vi "AODScanner.vi"() -> ()   [LabVIEW 2014]
uses:
  AODAcq/AODAcq.lvclass
  <vilib>/DAQmx/write.llb/DAQmx Write (Analog DBL 1Chan 1Samp).vi
  <vilib>/DAQmx/read.llb/DAQmx Read (Analog Wfm 1Chan NSamp).vi
  <vilib>/DAQmx/miscellaneous.llb/DAQmx Fill In Error Info.vi
  Motion Stabilization/GlobalVars.vi
  <vilib>/Utility/error.llb/Error Cluster From Error Code.vi
  <vilib>/rvi/errors/niLvFpgaAdjustHostInterfaceError.vi
  <vilib>/rvi/interface/nirviMethod/nirviMethod.xnode
  FPGA_Control/AODRef.ctl
  FPGA Bitfiles/AodScanner_FPGATarget_AODControl(FPGA)_TyJc9yYmyGA.lvbitx
  <vilib>/rvi/interface/nirviReadWriteControl/nirviReadWriteControl.xnode
  <vilib>/FPGAPlugInAG/PXIe-7965R/niLvFpga_ReadFifo_PXIe-7965R.vi
  <vilib>/rvi/errors/niLvFpgaMergeErrorWithErrorCode.vi
  NiFpgaLv.dll
panel:
  in  "Add":bool=TRUE
  out "ZOut um":dbl
  out "YOut um":dbl
  out "XOut um":dbl
  in  "Reset AOD Cum Offsets":bool
  out "Cum AOD Offset Z":dbl
  out "Cum AOD Offset X":dbl
  out "Cum AOD Offset Y":dbl
  in  "Noise Frequency (Hz)":dbl=0.1
  in  "Noise Amplitude (um)":dbl=3.0
  in  "Simulate Scanning Noise":bool
  in  "Invert Intensity":bool
  in  "AOD Feedback":bool
  out "XOut":i32
  out "ZOut":i32
  out "YOut":i32
  in  "Invert Z":bool=TRUE
  in  "Invert X":bool
  in  "Invert Y":bool=TRUE
  in  "Scan Offset X":dbl format="%#_13g"
  in  "Scan Offset Y":dbl format="%#_13g"
  in  "Scan Offset Z":dbl format="%#_13g"
  in  "Set AOD Scan Offset":bool
  out "globals_semaphore":T1
  out "Scan Settings Saved":T2
  out "y_scale":dbl
  out "x_scale":dbl
  out "Motion Points (Ch1)":u32
  in  "Per Cell Motion Analysis":bool
  in  "Sampling Structure":u16(ring) items=["Cube Vertices"]
  out "EventDone":bool
  in  "ForcePointScan":bool
  out "Selection":u32
  in  "ForceVolumeScan":bool
  out "Scan Settings (um) Saved":T2={"XStart"=-100, "XEnd"=100, "XNum"=250, "YStart"=-100, "YEnd"=100, "YNum"=250, "ZStart"=-30, "ZEnd"=70, "ZNum"=60}
  out "Motion FIFO":refnum<queue>
  out "Points_um":dbl[][](array[numeric])
  out "Stopped":bool
  in  "Power":dbl(slide)=2.5 min=0.0 max=5.0 step=0.1 scale=0.0..2.5
  in  "Debug":bool
  out "Number of Motion Planes":i32
  out "Motion Plane Centers":i32[][](array[numeric])
  in  "GridPoints":u16=10
  out "X-Y Motion Points":i32[][](array[numeric])
  out "Y-Z Motion Points":i32[][](array[numeric])
  out "error out":errorcluster
  out "error out 2":errorcluster
  in  "External Magnification":dbl=1.3
  in  "Matlab Server IP Address":string="10.21.16.18"
  in  "Matlab Server Shared Folder":string="c:\\temp"
  out "Histogram":dynamicdata(graph)
  out "ROIs":T3(array[cluster])
  out "Motion ROIs":T3(array[cluster])
  out "Waveform Chart":waveform(dbl)(graph)
  out "Ephys":bool
  in  "Points":i32[][](array[numeric])
  in  "Abort":bool
  out "ScanProgress":dbl(slide) scale=0.0..1.0
  in  "Simulated Motion Signal":bool
  in  "TraceElements":u32=10000
  out "Out Points":i32[][](array[numeric])
  in  "Tab Control":enum32{"Setup", "Volume", "Traces", "Motion"}(tab)
  in  "AOD Correction Threshold":dbl=0.25
  in  "AOD Feedback Gain":dbl=0.5
  in  "Average Motion Channels":bool
  in  "LoadAODVolume":bool
  in  "AOD Correction Refractory Time":dbl=1.0
  in  "Motor Correction Threshold":dbl=2.0 format="%#_13g"
  in  "Motion Tracking":bool
  in  "Auto Recentering":bool
  in  "XNum":i32=100
  in  "YNum":i32=100
  in  "Onset (fraction)":dbl=0.99 format="%#_13g"
  in  "Offset (fraction)":dbl=0.01 format="%#_13g"
  in  "Post Recentering Wait (ms)":u32=1000
  in  "Store Raw":bool
  in  "Disp Volume":bool=TRUE
  in  "Save Volume":bool
  in  "Ephys Acq":bool
  in  "Motion rate (Hz)":dbl=10.0
  in  "Scan Settings (um)":T2={"XStart"=-100, "XEnd"=100, "XNum"=250, "YStart"=-100, "YEnd"=100, "YNum"=250, "ZStart"=-30, "ZEnd"=70, "ZNum"=60}
  in  "Objective":enum16{"20x Olympus"}(ring)
  in  "Scan Time (s)":dbl=3000.0
  in  "Volume Reps":i32=1 min=1 max=10000
  in  "Volume Scan":bool
  in  "Points Scan":bool
  in  "Motion Channel To Analyze":i32=1 min=1 max=2
  in  "Motion Analysis":bool
  in  "Auto Motion Plane Params":T4={"Z Offset Per Box (um)"=3, "Box Size (um)"=16.0}
  in  "Mirror Ch1 Display":bool
  in  "ClearMotionCenters":bool
  in  "Point Centering":bool=TRUE
  in  "Recenter":bool caption="OK Button"
  out "Cells Selected":u32
  in  "Contrast":dbl(slide)=99.63636363636364 scale=98.0..100.0
  out "ImCh2":T5(plugin-control)
  out "ImCh1":T5(plugin-control)
  in  "Section":dbl min=0.0 max=59.0 step=1.0
  in  "Segment":bool
  out "Motion Increment":u32
  in  "Offset":dbl(slide)=0.010101010101010102 scale=0.0..1.0
  in  "ClearPoints":bool
  out "Total Motion Points":i32
  out "Number of Motion Volumes":i32
  out "Motion Ch1":T5(plugin-control)
  out "Ephys Signals":waveform(dbl)[](graph)
  in  "Baseline Offset":dbl
  in  "Decimate":bool
  in  "Spacing":dbl=100.0
  out "Traces":waveform(dbl)[](graph)
  in  "Down Rate":i32=500
  out "Elements In Traces Queue":i32
  out "Progress":dbl(slide) scale=0.0..1.0
  out "Scan Settings":T2
  in  "VolumeElements":u32=10000
  out "Recording File":path
  out "Objective Position":cluster{"X":dbl, "Y":dbl, "Z":dbl}
  out "Lens Magnification":i32=20
  out "Finished":bool
  out "Image samples remaining":u32
  out "Motion samples remaining":u32
  out "Temporal samples remaining":u32
  out "Raw samples remaining":u32
  in  "stop":bool
  out "AODAcq out":refnum<class "AODAcq.lvclass">
  out "Volume":bool
  out "Scan":bool
  in  "SweepSettings":bool
  out "Numeric":i32=299
  # "On"
  # "Off"
  # "um"
  # "sec"
  # "um"
  # "Motor"
  # "AOD+Motor"
  # "Off"
  # "On"
  # "Volume Resolution (points)"
  # "Behavior Pause"
  # "Off"
  # "On"
  # "Off"
  # "On"
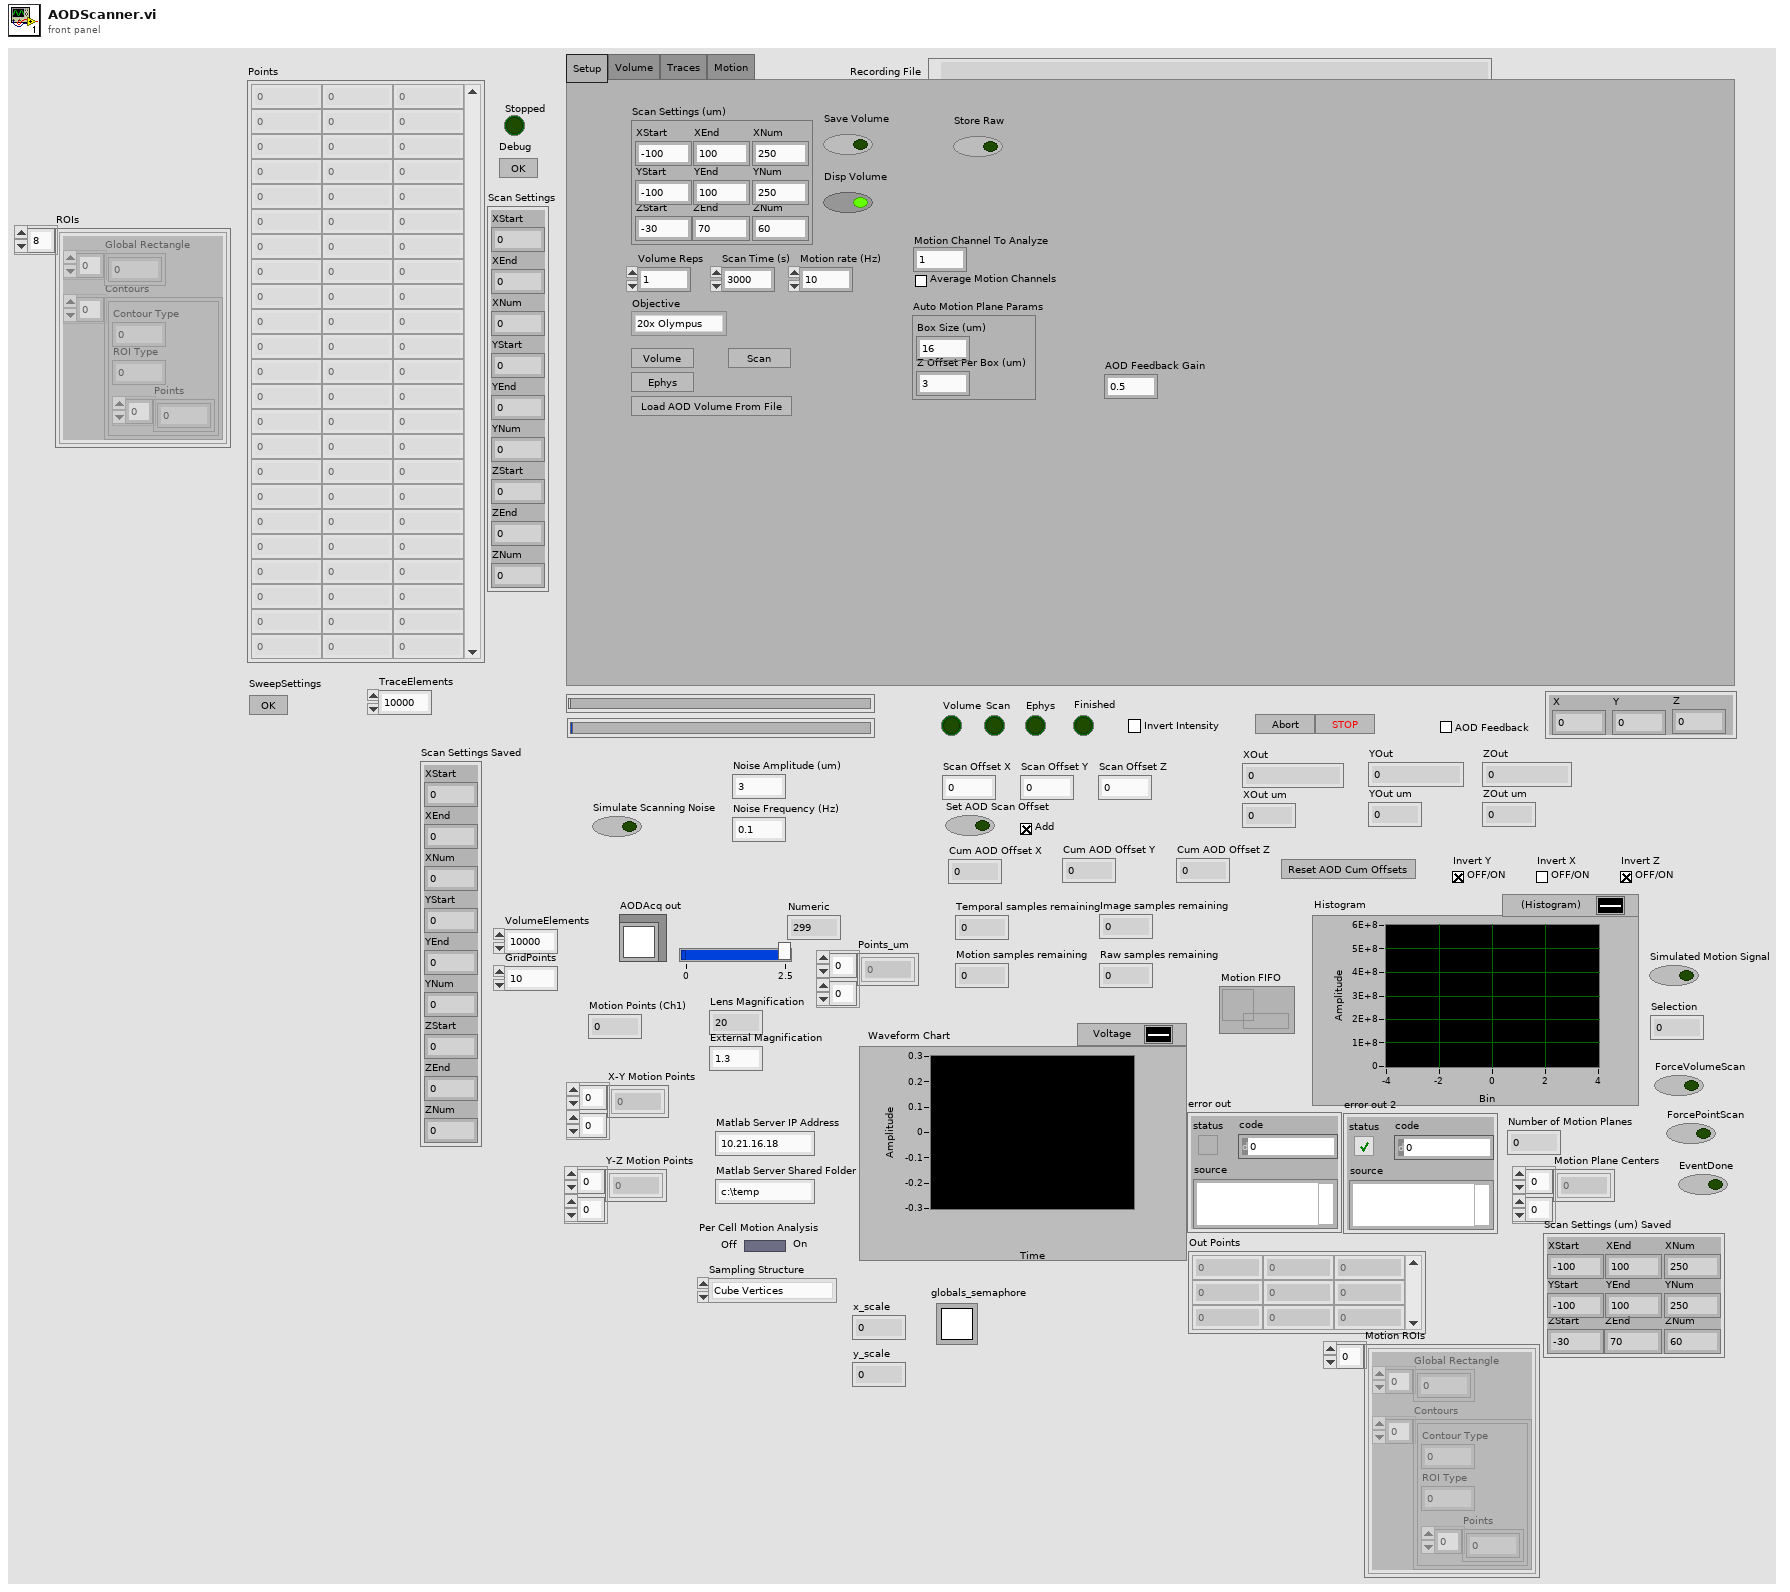
[diagram p1: front panel]
types:
  T1 = typedef "Semaphore RefNum" = refnum<k1>
  T2 = cluster{"XStart":i32, "XEnd":i32, "XNum":i32, "YStart":i32, "YEnd":i32, "YNum":i32, "ZStart":i32, "ZEnd":i32, "ZNum":i32}
  T3 = cluster{"Global Rectangle":i32[], "Contours":cluster{"Contour Type":u32, "ROI Type":u32, "Points":i32[]}[]}[]
  T4 = cluster{"Z Offset Per Box (um)":i32, "Box Size (um)":dbl}
  T5 = typedef "IMAQ Image.ctl" = refnum<image>
  T6 = cluster{"gridsize":u16, "data":i32[][], "coordinates":i32[][], "settings":i32[], "settings_um":i32[], "needsreference":bool}
  T7 = typedef "Image Type" = u32
  T8 = cluster{"Global Rectangle":i32[], "Contours":cluster{"Contour Type":u32, "ROI Type":u32, "Points":i32[]}[]}
  T9 = enum16{"big-endian, network order", "native, host order", "little-endian"}
  T10 = enum16{"open", "replace", "create", "open or create", "replace or create", "replace or create with confirmation"}
  T11 = cluster{"queue out":refnum<queue>, "queue out":refnum<queue>, "queue out":refnum<queue>, "queue out":refnum<queue>}
  T12 = typedef "AODRef.ctl" = refnum<k20>
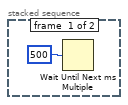
[diagram p2: hidden frame]
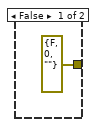
[diagram p4: hidden frame]
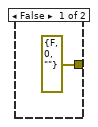
[diagram p5: hidden frame]
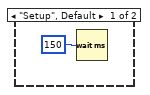
[diagram p6: hidden frame]
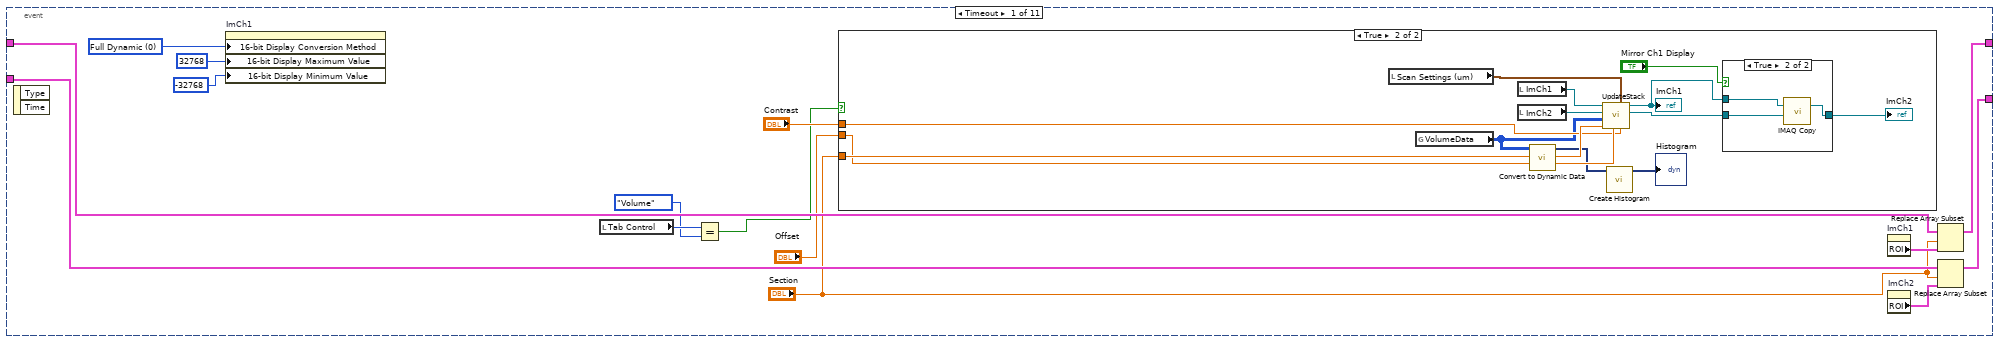
[diagram p8: hidden frame]
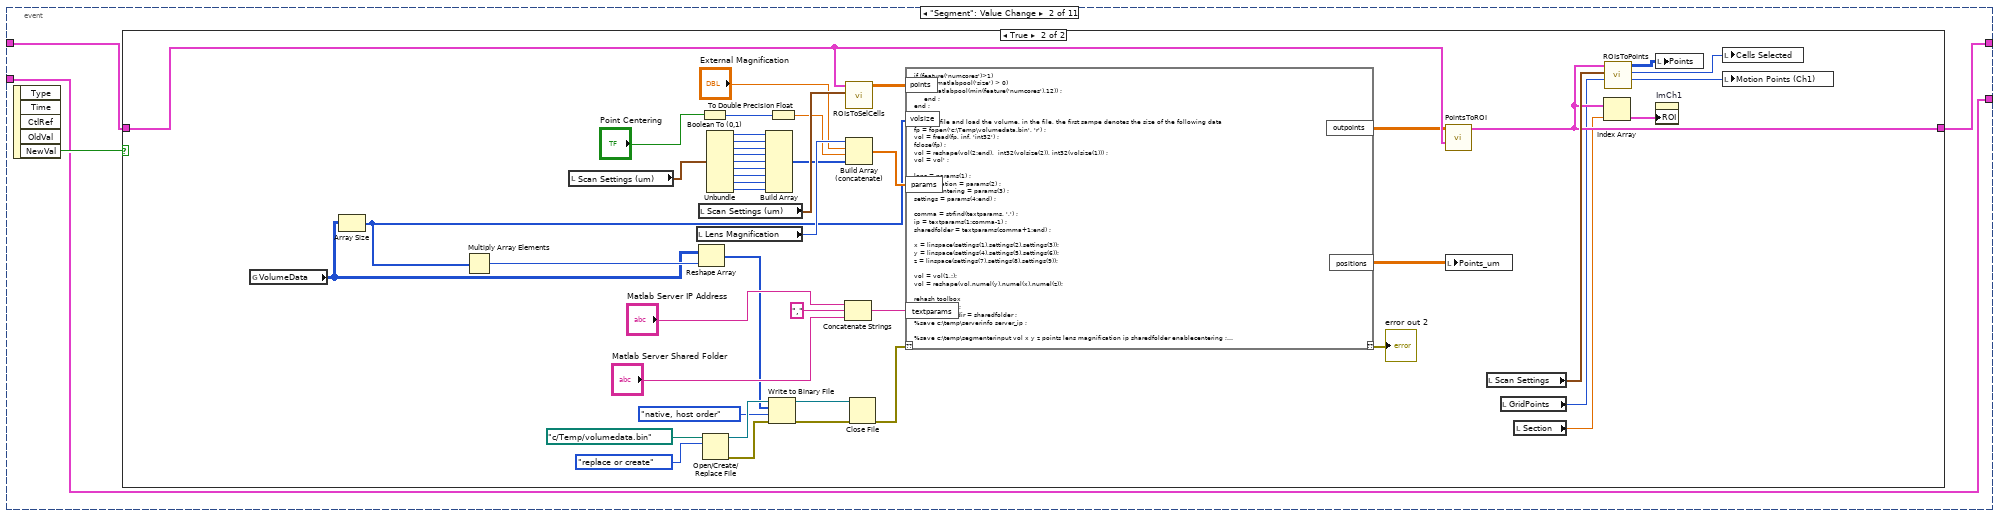
[diagram p11: hidden frame]
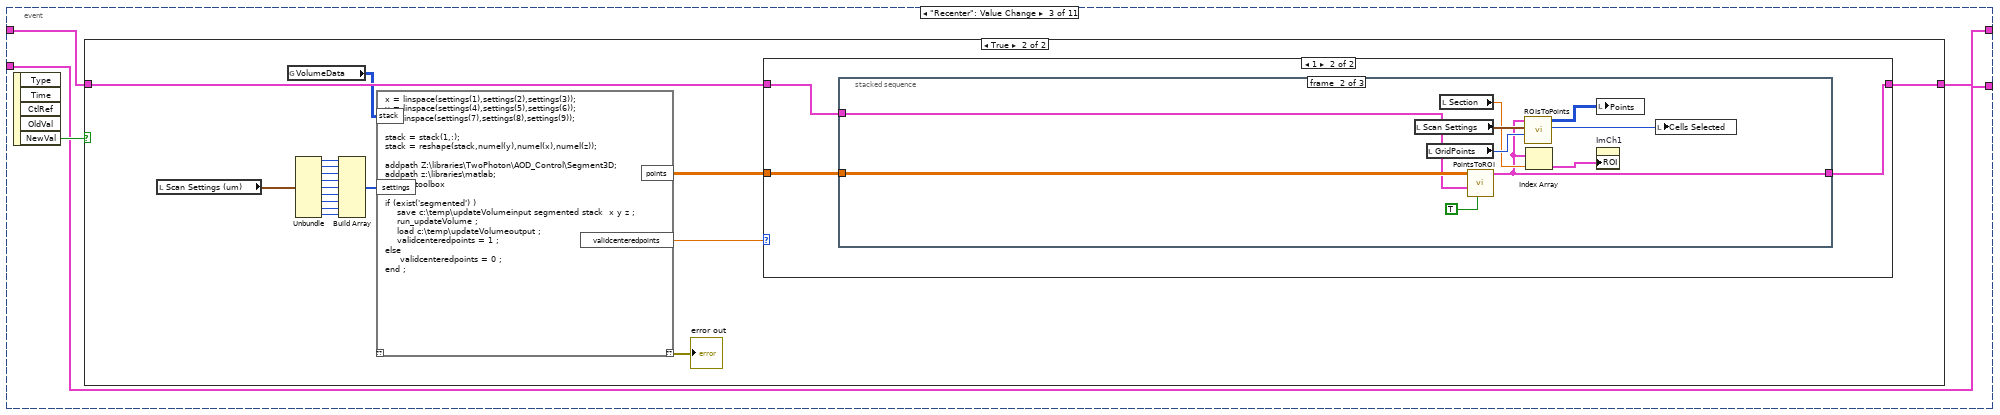
[diagram p13: hidden frame]
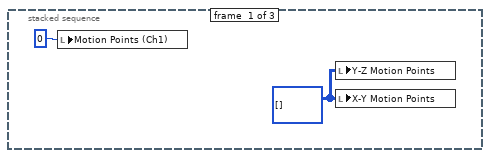
[diagram p16: hidden frame]
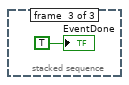
[diagram p17: hidden frame]
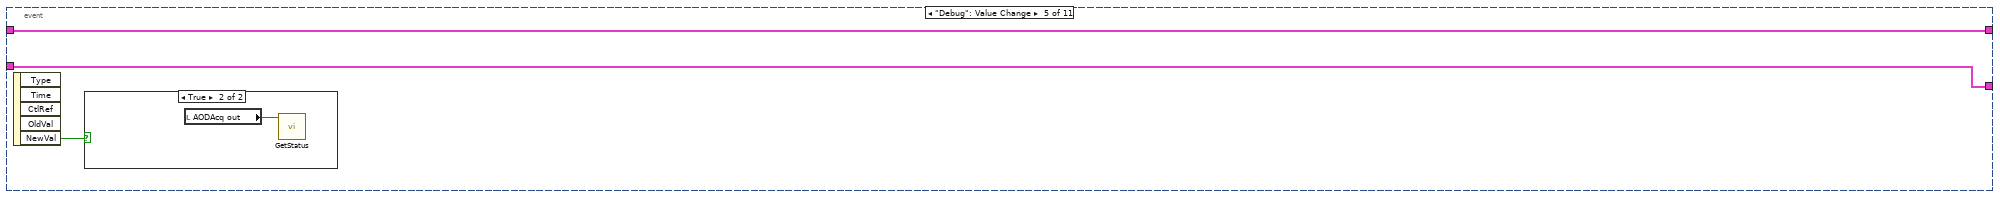
[diagram p19: hidden frame]
diagram:
  w11 = FALSE ("ForceVolumeScan")
  w27 = 100 ("max queue size (-1, unlimited)")
  w32 = T7 2 items=["Grayscale (U8)", "Grayscale (I16)", "Grayscale (SGL)", "Complex (CSG)", "RGB (U32)", "HSL (U32)", "RGB (U64)", "Grayscale (U16)"] ("Image Type")
  w9 = waveform(i32)[] []
  w42 = T7 0 items=["Grayscale (U8)", "Grayscale (I16)", "Grayscale (SGL)", "Complex (CSG)", "RGB (U32)", "HSL (U32)", "RGB (U64)", "Grayscale (U16)"] ("Image Type")
  w18 = T8 {"Global Rectangle"=[], "Contours"=[]} ("ROI")
  w52 = refnum<k21> "AOD Gain"  # DAQmx Global Channel
  n1 = local read "Scan Settings (um)"() -> (w46:T2)
  n2 = local write "ForceVolumeScan"(w11) -> ()
  n3 = local write "ForcePointScan"(w11) -> ()
  n4 = local write "Stopped"(FALSE ("Stopped")) -> ()
  n5 = local write "Stopped"(FALSE ("Stopped")) -> ()
  n6 = global write "GlobalVars.vi" "VI Open"(FALSE ("VI Open")) -> ()
  n7 = local write "Tab Control"(enum32{"Setup", "Volume", "Traces", "Motion"}."Setup" ("Tab Control")) -> ()
  n8 = Obtain Notifier(name (unnamed)="GoMove", notification data type="") -> (notifier out=w2:refnum<notifier>)  [unwired: 2 in, 2 out]
  n9 = Reciprocal(x="Motion rate (Hz)") -> (1/x=w20:dbl)
  n10 = global write "GlobalVars.vi" "Sampling Interval (sec)"(w20) -> ()
  n11 = global write "GlobalVars.vi" "GoMove Notifier"(w2) -> ()
  n12 = call <vilib>:"DAQmx Create Task.vi"("global virtual channels"=w52) -> ("task out"=w51:refnum<k21>, "error out"=w50:errorcluster)  [unwired: 4 in, 9 out]
  n13 = call "IMAQ Create"("Image Name"="Im1", "Image Type"=w42) -> ("New Image"=w54:T5)  [unwired: 3 in, 1 out]
  n14 = call "IMAQ Create"("Image Name"="Im2", "Image Type"=w42) -> ("New Image"=w53:T5)  [unwired: 3 in, 1 out]
  n15 = Unbundle By Name(w46) -> ("ZNum"=w17:i32)
  n16 = call "IMAQ Create"("Image Name"="Mot1", "Image Type"=w32) -> ("New Image"=→"Motion Ch1":T5)  [unwired: 3 in, 1 out]
  n17 = while {
    tunnel: w51 -> [w63]
    tunnel: w50 -> [w62]
    tunnel: [w61] -> w49
    tunnel: [w60] -> w48
    stop <- w59 stop-if-true
    n18 = Wait (ms)(milliseconds to wait=u32 1000) -> ()  [unwired: 1 out]
    n19 = local read "Stopped"() -> (w59:bool)
    n20 = call-poly <vilib>:"DAQmx Write.vi"("task/channels in"=w63, "data"="Power", "error in"=w62) -> ("task out"=w61:refnum<k21>, "error out"=w60:errorcluster)  [unwired: 10 in, 1 out]
  }
  n21 = local write "ImCh1"(w54) -> ()
  n22 = local write "ImCh2"(w53) -> ()
  n23 = Obtain Queue(max queue size (-1, unlimited)=w27, element data type=waveform(i32)[] []) -> (queue out=w38:refnum<queue>)  [unwired: 3 in, 2 out]
  n24 = Obtain Queue(max queue size (-1, unlimited)=w27, element data type=waveform(dbl)[] []) -> (queue out=w39:refnum<queue>)  [unwired: 3 in, 2 out]
  n25 = Obtain Queue(max queue size (-1, unlimited)=w27, element data type=w9) -> (queue out=w37:refnum<queue>)  [unwired: 3 in, 2 out]
  n26 = Obtain Queue(element data type=w9) -> (queue out=w8:refnum<queue>)  [unwired: 4 in, 2 out]
  n27 = call <vilib>:"Obtain Semaphore Reference.vi"("name (unnamed)"="globals") -> ("error out"=w5:errorcluster, "semaphore"=w6:T1)  [unwired: 4 in, 1 out]
  "globals_semaphore" <- w6
  n28 = Obtain Queue(name (unnamed)="Motion FIFO", element data type=0) -> (queue out=w13:refnum<queue>)  [unwired: 3 in, 2 out]
  "Motion FIFO" <- w13
  n29 = Obtain Queue(max queue size (-1, unlimited)=100, name (unnamed)="MotionAnalysis", element data type=T6 {"gridsize"=0, "data"=[], "coordinates"=[], "settings"=[], "settings_um"=[], "needsreference"=FALSE}) -> (queue out=w1:refnum<queue>)  [unwired: 2 in, 2 out]
  n30 = Decrement(x=w17) -> (x-1=w41:i32)
  n31 = Initialize Array(w18, w17) -> (w45:T3)
  n32 = Initialize Array(w18, w17) -> (w16:T3)
  n33 = while {
    shift-right: [w66] -> _
    shift-left: w45 -> [w70]
    shift-right: [w65] -> _
    shift-left: w16 -> [w67]
    stop <- w68 stop-if-true
    n34 = event shown="[3] \"Invert Intensity\": Value Change" {
      selector: _ -> [_ _ _ _ _ _ _ _ _ _ _]
      dyn-events: _ -> [_ _ _ _ _ _ _ _ _ _ _]
      timeout: 200 -> [_ _ _ _ _ _ _ _ _ _ _]
      tunnel: w70 -> [w84 w105 w156 w195 w202 w211 w239 w240 w253 w257 w269]
      tunnel: [w85 w104 w157 w195 w202 w211 w236 w240 w252 w258 w269] -> w66
      tunnel: [w72 w103 w155 w194 w201 w206 w228 w241 w249 w256 w270] -> w65
      tunnel: w67 -> [w75 w103 w155 w194 w201 w206 w228 w246 w251 w256 w268]
      event Timeout {
        w80 = u32 0 items=["Full Dynamic", "Downshift", "Given Range", "90% Dynamic", "Given Percent Range"] ("16-bit Display Mapping:Conversion Method")
        n35 = event-data() -> ()  [unwired: 1 in, 2 out]
        n36 = property on="ImCh1" class="ImageControl"("16-bit Display Conversion Method"=w80, "16-bit Display Maximum Value"=32768 ("16-bit Display Mapping:Maximum Value"), "16-bit Display Minimum Value"=-32768 ("16-bit Display Mapping:Maximum Value")) -> ()  [unwired: 2 in, 2 out]
        n37 = local read "Tab Control"() -> (w82:enum32{"Setup", "Volume", "Traces", "Motion"})
        n38 = Equal?(x=w82, y=enum32{"Setup", "Volume", "Traces"}."Volume") -> (x = y?=w71:bool)
        n39 = case shown="True" w71 {
          tunnel: "Section" -> [_ w95]
          tunnel: "Offset" -> [_ w94]
          tunnel: "Contrast" -> [_ w93]
          frame False {
          }
          frame True {
            n40 = local read "Scan Settings (um)"() -> (w96:T2)
            n41 = global read "GlobalVars.vi" "VolumeData"() -> (w86:i32[][])
            n42 = local read "ImCh1"() -> (w98:T5)
            n43 = local read "ImCh2"() -> (w97:T5)
            n44 = call "Convert to Dynamic Data"("2D Array"=w86) -> ("Dynamic Data Type"=w92:dynamicdata)  [unwired: 3 in]
            n45 = call "UpdateStack.vi"("Contrast"=w93, "Scan Settings"=w96, "Offset"=w94, "Section"=w95, "ImData"=w86, "Im2 2"=w97, "Im1 In"=w98) -> ("Im2 Out"=w87:T5, "Im1 Out"=w89:T5)  [unwired: 3 in]
            "ImCh1" <- w89
            n46 = call "Create Histogram"("Signal"=w92) -> ("Histogram"=→"Histogram":dynamicdata)  [unwired: 9 in, 1 out]
            n47 = case shown="True" "Mirror Ch1 Display" {
              tunnel: w89 -> [_ w101]
              tunnel: [w99 w100] -> w88
              tunnel: w87 -> [w99 w102]
              frame False {
              }
              frame True {
                n48 = call "IMAQ Copy"("Image Dst"=w102, "Image Src"=w101) -> ("Image Dst Out"=w100:T5)  [unwired: 4 in, 1 out]
              }
            }
            "ImCh2" <- w88
          }
        }
        n49 = property on="ImCh1" class="ImageControl"() -> ("ROI"=w83:T8)  [unwired: 2 in, 2 out]
        n50 = property on="ImCh2" class="ImageControl"() -> ("ROI"=w74:T8)  [unwired: 2 in, 2 out]
        n51 = Replace Array Subset(array=w84, new element=w83, index="Section") -> (w85:T3)
        n52 = Replace Array Subset(array=w75, new element=w74, index="Section") -> (w72:T3)
      }
      event "Segment": Value Change {
        n53 = event-data() -> ("NewVal"=w106:bool)  [unwired: 1 in, 4 out]
        n54 = case shown="True" w106 {
          tunnel: w105 -> [w107 w137]
          tunnel: [w107 w141] -> w104
          frame False {
          }
          frame True {
            n55 = global read "GlobalVars.vi" "VolumeData"() -> (w108:i32[][])
            n56 = Array Size(array=w108) -> (size(s)=w110:i32[])
            n57 = Multiply Array Elements(1:w110) -> (0:w117:i32)
            n58 = local read "Scan Settings (um)"() -> (w154:T2)
            n59 = local read "Lens Magnification"() -> (w133:i32)
            n60 = local read "Scan Settings (um)"() -> (w135:T2)
            n61 = Reshape Array(w108, w117) -> (w115:i32[])
            n62 = Boolean To (0,1)(Boolean="Point Centering") -> (0, 1=w138:i16)
            n63 = Open/Create/Replace File(file path (use dialog)=path "c:/Temp/volumedata.bin", operation (0:open)=T10."replace or create") -> (refnum out=w116:refnum<file>, error out=w114:errorcluster)  [unwired: 4 in, 1 out]
            n64 = Unbundle(w154) -> ("XStart"=w153:i32, "XEnd"=w152:i32, "XNum"=w151:i32, "YStart"=w150:i32, "YEnd"=w149:i32, "YNum"=w148:i32, "ZStart"=w147:i32, "ZEnd"=w146:i32, "ZNum"=w145:i32)
            n65 = Build Array(w153, w152, w151, w150, w149, w148, w147, w146, w145) -> (w127:i32[])
            n66 = Write to Binary File(file (use dialog)=w116, data=w115, error in=w114, 9:T9."native, host order" ("byte order (0:big-endian, network order)")) -> (refnum out=w112:refnum<file>, error out=w113:errorcluster)  [unwired: 2 in, 1 out]
            n67 = To Double Precision Float(number=w138) -> (double precision float=w131:dbl)
            n68 = Concatenate Strings("Matlab Server IP Address", "," ("string"), "Matlab Server Shared Folder") -> (w122:string)
            n69 = call "ROIsToSelCells.vi"("Scan Settings"=w135, "ROI"=w137) -> ("Points_um"=w134:dbl[][])  [unwired: 8 in, 1 out]
            n70 = Build Array (concatenate)(w133, "External Magnification", w131, w127) -> (w126:dbl[])
            n71 = Close File(refnum=w112, error in=w113) -> (error out=w111:errorcluster)  [unwired: 1 out]
            n72 = script code="if (feature('numcores')>1)\n     if (~matlabpool('size') > 0)\n         matlabpool(min(feature('numcores'),12)) ;\n     end ;\nend ;\n\n% open file and load the volume, in the file, the first sampe denotes the size of the following data\nfp = fopen('c:\\Temp\\volumedata.bin', 'r') ;\nvol = fread(fp, inf, 'int32') ;\nfclose(fp) ;\nvol = reshape(vol(2:end),  int32(volsize(2)), int32(volsize(1))) ;\nvol = vol' ;\n\nlens = params(1) ;\nmagnification = params(2) ;\nenablecentering = params(3) ;\nsettings = params(4:end) ;\n\ncomma = strfind(textparams, ',') ;\nip = textparams(1:comma-1) ;\nsharedfolder = textparams(comma+1:end) ;\n\nx = linspace(settings(1),settings(2),settings(3));\ny = linspace(settings(4),settings(5),settings(6));\nz = linspace(settings(7),settings(8),settings(9));\n\nvol = vol(1,:);\nvol = reshape(vol,numel(y),numel(x),numel(z));\n\nrehash toolbox\nserver_ip = ip ;\nserver_shareddir = sharedfolder ;\n%save c:\\temp\\serverinfo server_ip ;\n\n%save c:\\temp\\segmenterinput vol x y z points lens magnification ip sharedfolder enablecentering ;\n%remote_run_segmenter ;\nseg = aod.Segmenter(vol, x, y, z, points, lens, magnification, ip, sharedfolder, enablecentering ) ;\nsegmented = SegmenterDisplay(seg) ;\n\nfilename = sprintf('%s\\\\seg.mat', sharedfolder) ;\nload(filename) ;\npoints = centered_coordinates;\npositions = points; % in microns\n\n% Need to convert points into indicies into the array\nfor i = 1:size(points,1)\n   [~,idx] = min(abs(points(i,1)-x)); points(i,1) = idx;\n   [~,idx] = min(abs(points(i,2)-y)); points(i,2) = idx;\n   [~,idx] = min(abs(points(i,3)-z)); points(i,3) = idx;\nend\noutpoints = points ;"("??"=w111, "params"=w126, "textparams"=w122, "points"=w134, "volsize"=w110) -> ("??"=→"error out 2":errorcluster, "outpoints"=w121:dbl[][], "positions"=w120:dbl[][])
            n73 = call "PointsToROI.vi"("Old ROIs"=w137, "Points"=w121) -> ("ROIs"=w141:T3)  [unwired: 9 in]
            n74 = local write "Points_um"(w120) -> ()
            n75 = local read "Scan Settings"() -> (w143:T2)
            n76 = local read "GridPoints"() -> (w136:u16)
            n77 = local read "Section"() -> (w140:dbl)
            n78 = Index Array(array=w141, index=w140) -> (element=w142:T8)
            n79 = call "ROIsToPoints.vi"("GridPoints"=w136, "Scan Settings"=w143, "ROI"=w141) -> ("Number of motion points"=w124:i32, "Number of points"=w144:i32, "Points"=w123:i32[][])  [unwired: 4 in, 2 out]
            n80 = local write "Points"(w123) -> ()
            n81 = property on="ImCh1" class="ImageControl"("ROI"=w142) -> ()  [unwired: 2 in, 2 out]
            n82 = local write "Cells Selected"(w144) -> ()
            n83 = local write "Motion Points (Ch1)"(w124) -> ()
          }
        }
      }
      event "Recenter": Value Change {
        n84 = event-data() -> ("NewVal"=w158:bool)  [unwired: 1 in, 4 out]
        n85 = case shown="True" w158 {
          tunnel: [w159 w163] -> w157
          tunnel: w156 -> [w159 w164]
          frame False {
          }
          frame True {
            n86 = local read "Scan Settings (um)"() -> (w165:T2)
            n87 = global read "GlobalVars.vi" "VolumeData"() -> (w160:i32[][])
            n88 = Unbundle(w165) -> ("XStart"=w176:i32, "XEnd"=w175:i32, "XNum"=w174:i32, "YStart"=w173:i32, "YEnd"=w172:i32, "YNum"=w171:i32, "ZStart"=w170:i32, "ZEnd"=w169:i32, "ZNum"=w168:i32)
            n89 = Build Array(w176, w175, w174, w173, w172, w171, w170, w169, w168) -> (w167:i32[])
            n90 = script code="x = linspace(settings(1),settings(2),settings(3));\ny = linspace(settings(4),settings(5),settings(6));\nz = linspace(settings(7),settings(8),settings(9));\n\nstack = stack(1,:);\nstack = reshape(stack,numel(y),numel(x),numel(z));\n\naddpath Z:\\libraries\\TwoPhoton\\AOD_Control\\Segment3D;\naddpath z:\\libraries\\matlab;\nrehash toolbox\n\nif (exist('segmented') )\n    save c:\\temp\\updateVolumeinput segmented stack  x y z ;\n    run_updateVolume ;\n    load c:\\temp\\updateVolumeoutput ;\n    validcenteredpoints = 1 ;\nelse\n     validcenteredpoints = 0 ;\nend ;"("stack"=w160, "settings"=w167) -> ("??"=→"error out":errorcluster, "points"=w166:dbl[][], "validcenteredpoints"=w162:dbl)  [unwired: 1 in]
            n91 = case shown="1" w162 {
              tunnel: w166 -> [_ w180]
              tunnel: w164 -> [w177 w179]
              tunnel: [w177 w178] -> w163
              frame 0, Default {
              }
              frame 1 {
                n92 = stacked-sequence {
                  tunnel: w180 -> [_ w192 _]
                  tunnel: w179 -> [_ w188 _]
                  tunnel: [_ w185 _] -> w178
                  frame #0 {
                    w181 = i32[][] [] ("Points")
                    n93 = local write "Motion Points (Ch1)"(u32 0 ("Number of Motion Points")) -> ()
                    n94 = local write "Y-Z Motion Points"(w181) -> ()
                    n95 = local write "X-Y Motion Points"(w181) -> ()
                  }
                  frame #1 {
                    n96 = local read "Scan Settings"() -> (w189:T2)
                    n97 = local read "GridPoints"() -> (w190:u16)
                    n98 = local read "Section"() -> (w186:dbl)
                    n99 = call "PointsToROI.vi"("Clear Motion Planes"=TRUE, "Old ROIs"=w188, "Points"=w192) -> ("ROIs"=w185:T3)  [unwired: 8 in]
                    n100 = call "ROIsToPoints.vi"("GridPoints"=w190, "Scan Settings"=w189, "ROI"=w185) -> ("Number of points"=w191:i32, "Points"=w184:i32[][])  [unwired: 4 in, 3 out]
                    n101 = Index Array(array=w185, index=w186) -> (element=w187:T8)
                    n102 = local write "Points"(w184) -> ()
                    n103 = property on="ImCh1" class="ImageControl"("ROI"=w187) -> ()  [unwired: 2 in, 2 out]
                    n104 = local write "Cells Selected"(w191) -> ()
                  }
                  frame #2 {
                    "EventDone" <- TRUE ("EventDone")
                  }
                }
              }
            }
          }
        }
      }
      event "Invert Intensity": Value Change {
        n105 = event-data() -> ("OldVal"=w198:bool, "NewVal"=w197:bool)  [unwired: 1 in, 4 out]
        n106 = Not Equal?(x=w198, y=w197) -> (x != y?=w196:bool)
        n107 = case shown="True" w196 {
          frame False {
          }
          frame True {
            n108 = global read "GlobalVars.vi" "VolumeData"() -> (w200:i32[][])
            n109 = Negate(x=w200) -> (-x=w199:i32[][])
            n110 = global write "GlobalVars.vi" "VolumeData"(w199) -> ()
          }
        }
      }
      event "Debug": Value Change {
        n111 = event-data() -> ("NewVal"=w203:bool)  [unwired: 1 in, 4 out]
        n112 = case shown="True" w203 {
          frame False {
          }
          frame True {
            n113 = local read "AODAcq out"() -> (w204:refnum<class "AODAcq.lvclass">)
            n114 = call-dynamic "GetStatus.vi"("AODAcq in"=w204) -> ()  [unwired: 8 in, 3 out]
          }
        }
      }
      event "Section": Value Change {
        n115 = event-data() -> ("NewVal"=w205:dbl)  [unwired: 1 in, 4 out]
        n116 = Index Array(array=w211, index=w205) -> (element=w212:T8)
        n117 = Index Array(array=w206, index=w205) -> (element=w207:T8)
        n118 = local read "Tab Control"() -> (w210:enum32{"Setup", "Volume", "Traces", "Motion"})
        n119 = property on="ImCh1" class="ImageControl"("ROI"=w212) -> ()  [unwired: 2 in, 2 out]
        n120 = property on="ImCh2" class="ImageControl"("ROI"=w207) -> ()  [unwired: 2 in, 2 out]
        n121 = Equal?(x=w210, y=enum32{"Setup", "Volume", "Traces"}."Volume") -> (x = y?=w208:bool)
        n122 = case shown="True" w208 {
          tunnel: w205 -> [_ w221]
          frame False {
          }
          frame True {
            n123 = local read "Scan Settings (um)"() -> (w220:T2)
            n124 = global read "GlobalVars.vi" "VolumeData"() -> (w213:i32[][])
            n125 = local read "Contrast"() -> (w218:dbl)
            n126 = local read "ImCh1"() -> (w222:T5)
            n127 = local read "ImCh2"() -> (w223:T5)
            n128 = local read "Offset"() -> (w219:dbl)
            n129 = call "UpdateStack.vi"("Contrast"=w218, "Scan Settings"=w220, "Offset"=w219, "Section"=w221, "ImData"=w213, "Im2 2"=w223, "Im1 In"=w222) -> ("Im2 Out"=w216:T5, "Im1 Out"=w217:T5)  [unwired: 3 in]
            n130 = local read "Mirror Ch1 Display"() -> (w214:bool)
            n131 = local write "ImCh1"(w217) -> ()
            n132 = case shown="True" w214 {
              tunnel: w217 -> [_ w226]
              tunnel: [w224 w225] -> w215
              tunnel: w216 -> [w224 w227]
              frame False {
              }
              frame True {
                n133 = call "IMAQ Copy"("Image Dst"=w227, "Image Src"=w226) -> ("Image Dst Out"=w225:T5)  [unwired: 4 in, 1 out]
              }
            }
            n134 = local write "ImCh2"(w215) -> ()
          }
        }
      }
      event "GridPoints": Value Change; "ImCh1": Mouse Up {
        n135 = event-data() -> ()  [unwired: 1 in, 3 out]
        n136 = local read "Section"() -> (w237:dbl)
        n137 = property on="ImCh1" class="ImageControl"() -> ("ROI"=w238:T8)  [unwired: 2 in, 2 out]
        n138 = local read "Scan Settings"() -> (w235:T2)
        n139 = Replace Array Subset(array=w239, new element=w238, index=w237) -> (w236:T3)
        n140 = call "ROIsToPoints.vi"("GridPoints"="GridPoints", "Scan Settings"=w235, "ROI"=w236) -> ("X-Y Motion Points"=→"X-Y Motion Points":i32[][], "Number of motion points"=→"Motion Points (Ch1)":i32, "Number of points"=→"Cells Selected":i32, "Points"=w233:i32[][], "Y-Z Motion Points"=→"Y-Z Motion Points":i32[][])  [unwired: 4 in]
        n141 = local write "Points"(w233) -> ()
      }
      event "ImCh2": Mouse Up {
        n142 = event-data() -> ()  [unwired: 1 in, 3 out]
        n143 = local read "Section"() -> (w247:dbl)
        n144 = property on="ImCh2" class="ImageControl"() -> ("ROI"=w248:T8)  [unwired: 2 in, 2 out]
        n145 = local read "Scan Settings"() -> (w245:T2)
        n146 = local read "GridPoints"() -> (w244:u16)
        n147 = Replace Array Subset(array=w246, new element=w248, index=w247) -> (w241:T3)
        n148 = call "ROIsToPoints.vi"("GridPoints"=w244, "Scan Settings"=w245, "ROI"=w241) -> ("Number of points"=→"Number of Motion Planes":i32, "Points"=→"Motion Plane Centers":i32[][])  [unwired: 4 in, 3 out]
      }
      event "Scan Settings (um).ZNum": Value Change {
        n149 = event-data() -> ("NewVal"=w250:i32)  [unwired: 1 in, 4 out]
        n150 = Decrement(x=w250) -> (x-1=w254:i32)
        n151 = property on="Section" class="DigNum (strict)"("Maximum"=w254, "Minimum"=0.0 ("Data Entry Limits:Minimum")) -> ()  [unwired: 2 in, 2 out]
        n152 = Reshape Array(w253, w250) -> (w252:T3)
        n153 = Reshape Array(w251, w250) -> (w249:T3)
      }
      event "ClearPoints": Value Change {
        n154 = event-data() -> ("NewVal"=w259:bool)  [unwired: 1 in, 4 out]
        n155 = case shown="True" w259 {
          tunnel: [w260 w267] -> w258
          tunnel: w257 -> [w260 _]
          frame False {
          }
          frame True {
            w261 = u32 0 ("Number of Motion Points")
            w262 = i32[][] [] ("Points")
            w266 = T8 {"Global Rectangle"=[], "Contours"=[]} ("ROI")
            n156 = local write "Points"(w262) -> ()
            n157 = local write "Points_um"(dbl[][] [] ("Points_um")) -> ()
            n158 = local write "Cells Selected"(w261) -> ()
            n159 = local write "Motion Points (Ch1)"(w261) -> ()
            n160 = local read "Scan Settings"() -> (w265:T2)
            n161 = local write "Y-Z Motion Points"(w262) -> ()
            n162 = local write "X-Y Motion Points"(w262) -> ()
            n163 = property on="ImCh1" class="ImageControl"("ROI"=w266) -> ()  [unwired: 2 in, 2 out]
            n164 = Unbundle By Name(w265) -> ("ZNum"=w264:i32)
            n165 = Initialize Array(w266, w264) -> (w267:T3)
          }
        }
      }
      event "ClearMotionCenters": Value Change {
        n166 = event-data() -> ("NewVal"=w271:bool)  [unwired: 1 in, 4 out]
        n167 = case shown="True" w271 {
          tunnel: [w272 w273] -> w270
          tunnel: w268 -> [w272 _]
          frame False {
          }
          frame True {
            w274 = T8 {"Global Rectangle"=[], "Contours"=[]} ("ROI")
            n168 = local read "Scan Settings"() -> (w276:T2)
            n169 = property on="ImCh2" class="ImageControl"("ROI"=w274) -> ()  [unwired: 2 in, 2 out]
            n170 = Unbundle By Name(w276) -> ("ZNum"=w275:i32)
            n171 = Initialize Array(w274, w275) -> (w273:T3)
          }
        }
      }
    }
    "ROIs" <- w66
    "Motion ROIs" <- w65
    n172 = local read "Stopped"() -> (w68:bool)
  }
  n173 = global write "GlobalVars.vi" "MotionAnalysis"(w1) -> ()
  n174 = property on="Section" class="DigNum (strict)"("Increment"=1.0 ("Data Entry Limits:Increment"), "Maximum"=w41, "Minimum"=0.0 ("Data Entry Limits:Minimum")) -> ()  [unwired: 2 in, 2 out]
  n175 = Bundle("queue out"=w38, "queue out"=w39, "queue out"=w37, "queue out"=w8) -> (w36:T11)  [unwired: 1 in]
  n176 = call-dynamic "FpgaInit.vi"("AODAcq in"=refnum<class "AODAcq.lvclass"> refnum ("AODAcq.lvclass")) -> ("error out"=w30:errorcluster, "AODAcq out"=w29:refnum<class "AODAcq.lvclass">)  [unwired: 9 in]
  n177 = call <vilib>:"DAQmx Clear Task.vi"("task in"=w49, "error in"=w48) -> ()  [unwired: 13 in, 1 out]
  n178 = Unbundle(w36) -> ("queue out"=w35:refnum<queue>)  [unwired: 3 out]
  n179 = while {
    shift-right: [w288] -> _
    shift-left: w29 -> [w317]
    tunnel: w36 -> [w307]
    tunnel: w30 -> [w316]
    tunnel: ["stop"] -> w21
    tunnel: w1 -> [w309]
    tunnel: w13 -> [w308]
    tunnel: w6 -> [w280]
    tunnel: w5 -> [w279]
    i -> [w310]
    stop <- "stop" stop-if-true
    n180 = call <vilib>:"Acquire Semaphore.vi"("error in (no error)"=w279, "semaphore"=w280) -> ("error out"=w283:errorcluster, "semaphore out"=w284:T1)  [unwired: 3 in, 1 out]
    n181 = Unbundle(w307) -> ("queue out"=w306:refnum<queue>, "queue out"=w305:refnum<queue>, "queue out"=w304:refnum<queue>, "queue out"=w290:refnum<queue>)
    n182 = Flush Queue(queue=w306) -> ()  [unwired: 1 in, 3 out]
    n183 = Flush Queue(queue=w305) -> ()  [unwired: 1 in, 3 out]
    n184 = Flush Queue(queue=w304) -> ()  [unwired: 1 in, 3 out]
    n185 = Flush Queue(queue=w290) -> ()  [unwired: 1 in, 3 out]
    n186 = case shown="True" TRUE {
      tunnel: w284 -> [w325 w327]
      tunnel: w283 -> [w324 w326]
      tunnel: [w325 w327] -> w282
      tunnel: [w324 w326] -> w281
      frame False {
      }
      frame True {
        n187 = Get Date/Time In Seconds() -> (seconds since 1Jan1904=w332:timestamp)
        n188 = Initialize Array(0.0 ("element"), 3 ("dimension size")) -> (w328:dbl[])
        n189 = global write "GlobalVars.vi" "MovementSignal"(w328) -> ()
        n190 = shared-variable "My Computer\\SutterShared.lvlib\\TargetPosition"(w328) -> ()  [unwired: 1 in, 1 out]
        n191 = To Double Precision Float(number=w332) -> (double precision float=w331:dbl)
        n192 = global write "GlobalVars.vi" "AODPositionUpdateTime"(w331) -> ()
        n193 = global write "GlobalVars.vi" "MovementDetectionTime"(w331) -> ()
      }
    }
    n194 = Or(x="ForcePointScan", y="Points Scan") -> (x .or. y?=w298:bool)
    n195 = Or(x="ForceVolumeScan", y="Volume Scan") -> (x .or. y?=w302:bool)
    n196 = Build Array(w302, w298, "SweepSettings", "Ephys Acq", "LoadAODVolume") -> (w315:bool[])
    n197 = Boolean Array To Number(Boolean array=w315) -> (number=w277:u32)
    "Selection" <- w277
    n198 = case shown="2" w277 {
      tunnel: w317 -> [w439 w469 w552 w1144 w1167 w1187]
      tunnel: w316 -> [w446 w468 w595 w1143 _ w1188]
      tunnel: [w439 w450 w544 w1148 w1167 w1187] -> w289
      tunnel: [w446 w448 w568 w1147 w1166 w1186] -> w287
      tunnel: w307 -> [w443 w478 w611 _ w1169 _]
      tunnel: "Save Volume" -> [_ w477 _ _ _ _]
      tunnel: w309 -> [_ _ w540 _ _ _]
      tunnel: w308 -> [_ _ w580 _ _ _]
      frame 0, Default {
        w428 = 0 ("InOffset.X")
        n199 = call-dynamic "Read FPGA VI Reference.vi"("AODAcq in"=w439) -> ("FPGA VI Reference"=w429:T12)  [unwired: 8 in, 2 out]
        n200 = Unbundle(w443) -> ("queue out"=w442:refnum<queue>, "queue out"=w441:refnum<queue>, "queue out"=w440:refnum<queue>)  [unwired: 1 out]
        n201 = shared-variable "My Computer\\AODAcq.lvclass\\ReadFraction"(0.0 ("ReadFraction")) -> ()  [unwired: 1 in, 1 out]
        n202 = shared-variable "My Computer\\BehaviorShared.lvlib\\PauseBehavior"(FALSE ("PauseBehavior")) -> ()  [unwired: 1 in, 1 out]
        n203 = Wait (ms)(milliseconds to wait=u32 50) -> ()  [unwired: 1 out]
        n204 = Flush Queue(queue=w442) -> ()  [unwired: 1 in, 3 out]
        n205 = Flush Queue(queue=w441) -> ()  [unwired: 1 in, 3 out]
        n206 = Flush Queue(queue=w440) -> ()  [unwired: 1 in, 3 out]
        n207 = xnode "Invoke Method"("FPGA VI Reference In"=w429, "Number of Elements"=u32 0) -> ("Elements Remaining"=→"Motion samples remaining":u32)  [unwired: 2 in, 3 out]
        n208 = xnode "Invoke Method"("FPGA VI Reference In"=w429, "Number of Elements"=u32 0) -> ("Elements Remaining"=→"Image samples remaining":u32)  [unwired: 2 in, 3 out]
        n209 = xnode "Read/Write Control"("FPGA VI Reference In"=w429, "InOffset.X"=w428, "InOffset.Y"=w428, "InOffset.Z"=w428) -> ()  [unwired: 1 in, 2 out]
        n210 = xnode "Invoke Method"("FPGA VI Reference In"=w429, "Number of Elements"=u32 0) -> ("Elements Remaining"=→"Raw samples remaining":u32)  [unwired: 2 in, 3 out]
        n211 = xnode "Invoke Method"("FPGA VI Reference In"=w429, "Number of Elements"=u32 0) -> ("Elements Remaining"=→"Temporal samples remaining":u32)  [unwired: 2 in, 3 out]
        "Finished" <- FALSE ("Finished")
      }
      frame 1 {
        # "Volume imaging mode"
        n212 = local write "Volume Scan"(FALSE ("Volume")) -> ()
        n213 = case shown="\"20x Olympus\", Default" "Objective" {
          tunnel: [T2 {"XStart"=1460000, "XEnd"=1460000, "XNum"=1, "YStart"=1460000, "YEnd"=1460000, "YNum"=1, "ZStart"=700, "ZEnd"=700, "ZNum"=1} ("y")] -> w493
          tunnel: [20] -> w454
          frame "20x Olympus", Default {
          }
        }
        "Lens Magnification" <- w454
        n214 = call "GetObjectivePosition.vi"() -> ("output cluster"=w455:cluster{"X":dbl, "Y":dbl, "Z":dbl})  [unwired: 8 in, 3 out]
        "Objective Position" <- w455
        n215 = local write "Tab Control"(enum32{"Setup", "Volume", "Traces"}."Volume" ("Tab Control")) -> ()
        n216 = call-dynamic "Init.vi"("error in (no error)"=w468, "Channel"=i16 3, "AODAcq in"=w469) -> ("error out"=w467:errorcluster, "AODAcq out"=w466:refnum<class "AODAcq.lvclass">)  [unwired: 7 in]
        n217 = call-dynamic "Reset.vi"("error in (no error)"=w467, "AODAcq in"=w466) -> ("error out"=w458:errorcluster, "AODAcq out"=w459:refnum<class "AODAcq.lvclass">)  [unwired: 8 in]
        n218 = local read "ForceVolumeScan"() -> (w451:bool)
        n219 = Unbundle By Name("Scan Settings (um)") -> ("XNum"=w495:i32, "YNum"=w494:i32, "ZNum"=w463:i32)
        n220 = call-dynamic "Write Object Position.vi"("error in (no error)"=w458, "Object Position"=w455, "AODAcq in"=w459) -> ("error out"=w456:errorcluster, "AODAcq out"=w457:refnum<class "AODAcq.lvclass">)  [unwired: 7 in]
        n221 = Multiply(x=w493, y="Scan Settings (um)") -> (x*y=w452:T2)
        "Scan Settings" <- w452
        n222 = case shown="False" w451 {
          tunnel: "Scan Settings (um)" -> [w499 _]
          tunnel: w452 -> [w498 _]
          frame False {
            "Scan Settings (um) Saved" <- w499
            "Scan Settings Saved" <- w498
          }
          frame True {
          }
        }
        n223 = call-dynamic "Configure Volume.vi"("Save"=w477, "error in (no error)"=w456, "NumReps"="Volume Reps", "Scan Settings"=w452, "AODAcq in"=w457) -> ("error out"=w481:errorcluster, "AODAcq out"=w482:refnum<class "AODAcq.lvclass">)  [unwired: 5 in]
        n224 = Select(t=w463, s="Disp Volume", f=u32 1) -> (s? t:f=w462:u32)
        n225 = Compound Arithmetic op=MULTIPLY(w495, w494, w462) -> (w460:u32)
        n226 = call-dynamic "Start.vi"("error in (no error)"=w481, "AODAcq in"=w482) -> ("error out"=w473:errorcluster, "AODAcq out"=w475:refnum<class "AODAcq.lvclass">)  [unwired: 8 in]
        n227 = call-dynamic "Read Recording File.vi"("error in (no error)"=w473, "AcquistionObject in"=w475) -> ("error out"=w472:errorcluster, "Recording File"=→"Recording File":path, "AcquistionObject out"=w474:refnum<class "AODAcq.lvclass">)  [unwired: 7 in]
        n228 = call-dynamic "Read FPGA VI Reference.vi"("error in (no error)"=w472, "AODAcq in"=w474) -> ("error out"=w479:errorcluster, "FPGA VI Reference"=w485:T12, "AODAcq out"=w480:refnum<class "AODAcq.lvclass">)  [unwired: 7 in]
        n229 = Unbundle(w478) -> ("queue out"=w486:refnum<queue>, "queue out"=w483:refnum<queue>)  [unwired: 2 out]
        n230 = Initialize Array(0, 2 ("dimension size"), w460) -> (w492:i32[][])
        n231 = call-dynamic "Read Loop.vi"("error in (no error)"=w479, "ReadElements"="VolumeElements", "Queues"=w478, "AODAcq in"=w480) -> ("error out"=w449:errorcluster, "AODAcq out"=w450:refnum<class "AODAcq.lvclass">)  [unwired: 6 in]
        n232 = while {
          tunnel: w486 -> [w519]
          shift-right: [w503] -> _
          shift-left: w492 -> [w507]
          shift-right: [w516] -> _
          shift-left: 0 -> [w517]
          tunnel: w460 -> [w515]
          tunnel: 1000 ("timeout in ms (-1)") -> [w514]
          tunnel: w485 -> [w511]
          tunnel: w483 -> [w509]
          stop <- w512 stop-if-true
          n233 = Flush Queue(queue=w509) -> ()  [unwired: 1 in, 3 out]
          n234 = local read "Abort"() -> (w508:bool)
          n235 = xnode "Read/Write Control"("FPGA VI Reference In"=w511, "Control.Abort"=w508) -> ()  [unwired: 1 in, 2 out]
          n236 = Dequeue Element(queue=w519, timeout in ms (-1)=w514) -> (element=w518:waveform(i32)[], timed out?=w506:bool)  [unwired: 1 in, 2 out]
          n237 = shared-variable "My Computer\\AODAcq.lvclass\\ScanFraction"() -> (w510:dbl)  [unwired: 1 in, 1 out]
          n238 = shared-variable "My Computer\\AODAcq.lvclass\\ReadFraction"() -> (→"Progress":dbl)  [unwired: 1 in, 1 out]
          n239 = case shown="False" w506 {
            tunnel: w507 -> [w528 w537]
            tunnel: w518 -> [w527 _]
            tunnel: w517 -> [w526 w536]
            tunnel: [w525 w536] -> w516
            tunnel: [w524 w537] -> w504
            tunnel: w515 -> [w523 _]
            tunnel: [_ w535] -> w512
            frame False {
              n240 = for {
                tunnel: w528 -> [w532] mode=indexing
                tunnel: w527 -> [w534] mode=indexing
                tunnel: [w533] -> w524 mode=indexing
                tunnel: w526 -> [w530]
                tunnel: [w531] -> w525
                tunnel: w523 -> [_]
                n241 = Unbundle By Name(w534) -> ("Y"=w529:i32[])
                n242 = call "WraparoundUpdate.vi"("Data"=w529, "Location"=w530, "Accumulator"=w532) -> ("NewLocation"=w531:u32, "Accumulated"=w533:i32[])  [unwired: 7 in]
              }
            }
            frame True {
              n243 = local read "Finished"() -> (w535:bool)
            }
          }
          n244 = local write "ScanProgress"(w510) -> ()
          n245 = case shown="False" "Invert Intensity" {
            tunnel: w504 -> [w520 w522]
            tunnel: [w520 w521] -> w503
            frame False {
            }
            frame True {
              n246 = Negate(x=w522) -> (-x=w521:i32[][])
            }
          }
          n247 = global write "GlobalVars.vi" "VolumeData"(w503) -> ()
        }
        n248 = flat-sequence {
          tunnel: w449 -> [w500]
          tunnel: [FALSE] -> w476
          tunnel: [w500] -> w448
          frame #0 {
            n249 = local write "Finished"(TRUE ("Finished")) -> ()
          }
        }
        n250 = local write "Save Volume"(w476) -> ()
      }
      frame 2 {
        w549 = 3 ("dimension size")
        w550 = 0.0 ("element")
        w596 = i16 3  # Timestamp Timer Channel
        w573 = 300 ("timeout in ms (-1)")
        # "Point imaging mode"
        n251 = Flush Queue(queue=w580) -> (queue out=w579:refnum<queue>)  [unwired: 1 in, 2 out]
        n252 = global write "GlobalVars.vi" "Scanning"(TRUE ("Scanning")) -> ()
        n253 = local write "Points Scan"(FALSE ("Scan")) -> ()
        n254 = local write "Tab Control"(enum32{"Setup", "Volume", "Traces"}."Traces" ("Tab Control")) -> ()
        n255 = call-dynamic "Init.vi"("error in (no error)"=w595, "Channel"=w596, "AODAcq in"=w552) -> ("error out"=w591:errorcluster, "AODAcq out"=w588:refnum<class "AODAcq.lvclass">)  [unwired: 7 in]
        n256 = call "GetObjectivePosition.vi"() -> ("output cluster"=w587:cluster{"X":dbl, "Y":dbl, "Z":dbl})  [unwired: 8 in, 3 out]
        n257 = local read "Simulated Motion Signal"() -> (w569:bool)
        n258 = local read "Scan Settings (um)"() -> (w561:T2)
        n259 = local write "Objective Position"(w587) -> ()
        n260 = call-dynamic "Write Object Position.vi"("error in (no error)"=w591, "Object Position"=w587, "AODAcq in"=w588) -> ("error out"=w590:errorcluster, "AODAcq out"=w589:refnum<class "AODAcq.lvclass">)  [unwired: 7 in]
        n261 = local read "Cells Selected"() -> (w581:u32)
        n262 = local read "Scan Settings"() -> (w562:T2)
        n263 = call-dynamic "Reset.vi"("error in (no error)"=w590, "AODAcq in"=w589) -> ("error out"=w618:errorcluster, "AODAcq out"=w585:refnum<class "AODAcq.lvclass">)  [unwired: 8 in]
        n264 = case shown="True" w569 {
          tunnel: [dbl[][] [] w912] -> w577
          tunnel: [dbl[][] [] w910] -> w571
          tunnel: w562 -> [_ w916]
          tunnel: w561 -> [_ w915]
          frame False {
          }
          frame True {
            # "The volume is 250x250x60, so the scan settings are set to this"
            n265 = Cluster To Array(cluster=w916) -> (array=w914:i32[])
            n266 = Cluster To Array(cluster=w915) -> (array=w913:i32[])
            n267 = call "ReadTestData.vi"("settings_um"=w913, "settings_aod"=w914) -> ("coordinates"=w910:dbl[][], "linearvolume"=w911:dbl[][], "testdata"=w912:dbl[][])  [unwired: 7 in]
            n268 = global write "GlobalVars.vi" "VolumeData"(w911) -> ()
          }
        }
        n269 = local read "Motion Points (Ch1)"() -> (w556:u32)
        n270 = local read "Motion rate (Hz)"() -> (w563:dbl)
        n271 = local read "Motion ROIs"() -> (w566:T3)
        n272 = local read "GridPoints"() -> (w564:u16)
        n273 = call-dynamic "ConfigurePerCellMotionAnalysis.vi"("Scan Settings (um)"=w561, "Points Selected"=w581, "Scan Settings"=w562, "Sampling Structure"="Sampling Structure", "Per Cell Motion Analysis"="Per Cell Motion Analysis", "In Points"="Points", "AODAcq in"=w585) -> ("Additional Points"=w583:i32, "Out Points"=w565:i32[][])  [unwired: 1 in, 2 out]
        n274 = case shown="False" "Per Cell Motion Analysis" {
          tunnel: w581 -> [w974 w978]
          tunnel: w583 -> [_ w977]
          tunnel: [w974 w975] -> w576
          frame False {
          }
          frame True {
            n275 = Multiply(x=w978, y=w977) -> (x*y=w976:u32)
            n276 = Add(x=w978, y=w976) -> (x+y=w975:u32)
          }
        }
        n277 = call "AutoConfigureAdditionalMotionPlanes.vi"("Motion ROIs"=w566, "In Points"=w565, "Grid Points"=w564, "Motion Rate (Hz)"=w563, "Number of Motion Points"=w556, "Scan Settings"=w562, "Plane Params"="Auto Motion Plane Params", "Scan Settings (um)"=w561) -> ("X-Y Motion Points"=w554:i32[][], "Y-Z Motion Points"=w560:i32[][], "Out Points"=w559:i32[][], "Total Motion Points"=w558:i32, "Number of Motion Volumes"=→"Number of Motion Volumes":i32, "Motion Increment"=w557:i32)  [unwired: 4 in, 2 out]
        "Out Points" <- w559
        "Total Motion Points" <- w558
        n278 = local read "GridPoints"() -> (w606:u16)
        n279 = local write "X-Y Motion Points"(w554) -> ()
        n280 = local write "Motion Increment"(w557) -> ()
        n281 = local write "Y-Z Motion Points"(w560) -> ()
        n282 = Quotient & Remainder(x=w558, y=w606) -> (floor(x/y)=w607:i32)  [unwired: 1 out]
        n283 = Multiply(x="Scan Time (s)", y=50000.0) -> (x*y=w615:dbl)
        n284 = Decrement(x=w557) -> (x-1=w602:i32)
        n285 = Divide(x=w602, y=w557) -> (x/y=w601:dbl)
        n286 = Divide(x=w615, y=w576) -> (x/y=w604:dbl)
        n287 = Quotient & Remainder(x="TraceElements", y=w576) -> (floor(x/y)=w574:u32)  [unwired: 1 out]
        n288 = Unbundle(w611) -> ("queue out"=w575:refnum<queue>, "queue out"=w608:refnum<queue>)  [unwired: 2 out]
        n289 = Multiply(x=w601, y=w604) -> (x*y=w603:dbl)
        n290 = Multiply(x=w576, y=w574) -> (x*y=w612:u32)
        n291 = Initialize Array "Cumulative Motor Motion Signal"(w550, w549) -> (w551:dbl[])
        n292 = while {
          tunnel: w576 -> [w923]
          tunnel: w575 -> [w918]
          tunnel: w574 -> [w922]
          tunnel: w573 -> [w921]
          tunnel: 0 -> [w920]
          stop <- w919 continue-if-true
          n293 = Get Queue Status(queue=w918) -> (# elements in queue=→"Elements In Traces Queue":i32)  [unwired: 2 in, 7 out]
          n294 = Dequeue Element(queue=w918, timeout in ms (-1)=w921) -> (element=w925:waveform(i32)[])  [unwired: 1 in, 3 out]
          n295 = Divide(x=50000, y=w923) -> (x/y=w930:dbl)
          n296 = Divide(x=w930, y="Down Rate") -> (x/y=w932:dbl)
          n297 = Round To Nearest(number=w932) -> (nearest integer value=w928:dbl)
          n298 = In Range and Coerce(upper limit=w922, x=w928, lower limit=1.0) -> (coerced(x)=w926:dbl)  [unwired: 1 out]
          n299 = case shown="\"Traces\"" "Tab Control" {
            tunnel: w923 -> [_ w951]
            tunnel: w925 -> [_ w957]
            tunnel: w926 -> [_ w954]
            tunnel: w920 -> [_ w936]
            frame Default {
            }
            frame "Traces" {
              n300 = Index Array(array=w957, index=0) -> (element=w934:waveform(i32))
              n301 = local read "Invert Intensity"() -> (w935:bool)
              n302 = case shown="False" w935 {
                tunnel: w934 -> [w961 w963]
                tunnel: [w961 w962] -> w933
                frame False {
                }
                frame True {
                  n303 = Negate(x=w963) -> (-x=w962:waveform(i32))
                }
              }
              n304 = Add(x=w933, y="Baseline Offset") -> (x+y=w937:waveform(dbl))
              n305 = Unbundle By Name(w937) -> ("dt"=w959:dbl, "Y"=w956:dbl[])
              n306 = Multiply(x=w951, y=w959) -> (x*y=w958:dbl)
              n307 = Array Size(array=w956) -> (size(s)=w946:i32)
              n308 = Divide(x=w946, y=w951) -> (x/y=w950:dbl)
              n309 = feedback #1(w936) -> (w945:i32)
              n310 = Add(x=w946, y=w945) -> (x+y=w941:i32)
              n311 = feedback-in #1(w941) -> ()
              n312 = Reshape Array(w956, w950, w951) -> (w949:dbl[][])
              n313 = Less?(x=w941, y=50000) -> (x < y?=w939:bool)
              n314 = Transpose 2D Array(2D array=w949) -> (transposed array=w948:dbl[][])
              n315 = for {
                tunnel: w958 -> [w973]
                tunnel: w937 -> [w972]
                tunnel: [w971] -> w953 mode=indexing
                tunnel: w948 -> [w970] mode=indexing
                n316 = Bundle By Name(cluster=w972, "dt"=w973, "Y"=w970) -> (w971:waveform(dbl))
              }
              n317 = Select(t=1.0, s=w939, f=0.001 ("Baseline Rate")) -> (s? t:f=w942:dbl)
              n318 = case shown="True" "Decimate" {
                tunnel: "Spacing" -> [_ w969]
                tunnel: w954 -> [_ w968]
                tunnel: w953 -> [w964 w967]
                tunnel: [w964 w966] -> w952
                tunnel: w942 -> [_ w965]
                frame False {
                }
                frame True {
                  n319 = call "CleanupTraces.vi"("Baseline Rate"=w965, "Spacing"=w969, "decimating factor"=w968, "Traces in"=w967) -> ("Traces out"=w966:waveform(dbl)[])  [unwired: 7 in]
                }
              }
              "Traces" <- w952
            }
          }
          n320 = global read "GlobalVars.vi" "Scanning"() -> (w919:bool)
        }
        n321 = call-dynamic "Configure PointScan.vi"("AODAcq in"=w585, "Save"=TRUE ("Save Volume"), "Store Raw"="Store Raw", "Points"=w559, "GridSize"=w564, "Reps"=w603, "error in (no error)"=w618, "Motion Points"=w558, "Motion Increment"=w557) -> ("AODAcq out"=w609:refnum<class "AODAcq.lvclass">, "error out"=w610:errorcluster)  [unwired: 5 in]
        n322 = Initialize Array "Cumulative AOD Motion Signal"(w550, w549) -> (w548:dbl[])
        n323 = call-dynamic "Read FPGA VI Reference.vi"("error in (no error)"=w610, "AODAcq in"=w609) -> ("error out"=w600:errorcluster, "FPGA VI Reference"=w542:T12, "AODAcq out"=w546:refnum<class "AODAcq.lvclass">)  [unwired: 7 in]
        n324 = local read "Motion Analysis"() -> (w547:bool)
        n325 = call-dynamic "Start.vi"("error in (no error)"=w600, "AODAcq in"=w546) -> ("error out"=w598:errorcluster, "AODAcq out"=w599:refnum<class "AODAcq.lvclass">)  [unwired: 8 in]
        n326 = call-dynamic "Read Recording File.vi"("error in (no error)"=w598, "AcquistionObject in"=w599) -> ("error out"=w593:errorcluster, "Recording File"=w597:path, "AcquistionObject out"=w545:refnum<class "AODAcq.lvclass">)  [unwired: 7 in]
        n327 = case shown="True" w547 {
          tunnel: w551 -> [_ w627]
          tunnel: w542 -> [_ w619]
          tunnel: w548 -> [_ w626]
          tunnel: w545 -> [_ w625]
          tunnel: w540 -> [_ w620]
          frame False {
          }
          frame True {
            w624 = 0  # accumulated samples
            n328 = while "Add Position Noise To AOD Scanning" {
              tunnel: w619 -> [w664]
              stop <- w666 continue-if-true
              n329 = Reciprocal(x="Noise Frequency (Hz)") -> (1/x=w662:dbl)
              n330 = case shown="True" "Simulate Scanning Noise" {
                tunnel: w664 -> [_ w678]
                frame False {
                }
                frame True {
                  w674 = 0.5 ("y")
                  n331 = Random Number (0-1)() -> (number: 0 to 1=w677:dbl)
                  n332 = Random Number (0-1)() -> (number: 0 to 1=w676:dbl)
                  n333 = Random Number (0-1)() -> (number: 0 to 1=w675:dbl)
                  n334 = local read "Scan Settings (um)"() -> (w680:T2)
                  n335 = Subtract(x=w677, y=w674) -> (x-y=w673:dbl)
                  n336 = Subtract(x=w676, y=w674) -> (x-y=w671:dbl)
                  n337 = Subtract(x=w675, y=w674) -> (x-y=w670:dbl)
                  n338 = local read "Scan Settings"() -> (w679:T2)
                  n339 = Multiply(x=w673, y="Noise Amplitude (um)") -> (x*y=w669:dbl)
                  n340 = Multiply(x=w671, y="Noise Amplitude (um)") -> (x*y=w668:dbl)
                  n341 = Multiply(x=w670, y="Noise Amplitude (um)") -> (x*y=w667:dbl)
                  n342 = call "Add AOD Scanning Offsets.vi"("Scan Settings"=w679, "Scan Settings (um)"=w680, "Scan Offset Z"=w667, "Scan Offset Y"=w668, "Scan Offset X"=w669, "FPGA VI Reference"=w678) -> ()  [unwired: 6 in]
                }
              }
              n343 = Multiply(x=w662, y=1000.0) -> (x*y=w660:dbl)
              n344 = Wait (ms)(milliseconds to wait=w660) -> ()  [unwired: 1 out]
              n345 = global read "GlobalVars.vi" "Scanning"() -> (w666:bool)
            }
            n346 = while "Reset the AOD offsets after a motor movement in response to aggregated aod offsets reaching a threshold" {
              tunnel: w620 -> [w635]
              tunnel: w619 -> [w634]
              stop <- w636 stop-if-true
              n347 = local read "globals_semaphore"() -> (w633:T1)
              n348 = call <vilib>:"Acquire Semaphore.vi"("semaphore"=w633) -> ("error out"=w629:errorcluster, "semaphore out"=w632:T1)  [unwired: 4 in, 1 out]
              n349 = case shown="True" TRUE {
                tunnel: w635 -> [_ w644]
                tunnel: w634 -> [_ w643]
                tunnel: w632 -> [w638 w642]
                tunnel: [w638 w641] -> w630
                tunnel: w629 -> [w637 w640]
                tunnel: [w637 w639] -> w628
                frame False {
                }
                frame True {
                  n350 = global read "GlobalVars.vi" "Motor Movement Commant Sent"() -> (w647:bool)
                  n351 = global read "GlobalVars.vi" "Motor Movement Completed"() -> (w646:bool)
                  n352 = And(x=w647, y=w646) -> (x .and. y?=w645:bool)
                  n353 = case shown="True" w645 {
                    tunnel: w644 -> [_ w654]
                    tunnel: w643 -> [_ w653]
                    tunnel: [w649 w651] -> w641
                    tunnel: w642 -> [w649 w651]
                    tunnel: w640 -> [w648 w650]
                    tunnel: [w648 w650] -> w639
                    frame False {
                    }
                    frame True {
                      n354 = flat-sequence {
                        tunnel: w653 -> [w656]
                        tunnel: w654 -> [w659]
                        frame #0 {
                          w655 = 0 ("index")
                          n355 = local read "Scan Settings (um)"() -> (w658:T2)
                          n356 = local read "Scan Settings"() -> (w657:T2)
                          n357 = call "Set AOD Scanning Offsets.vi"("Scan Settings"=w657, "Scan Settings (um)"=w658, "Scan Offset Z"=w655, "Scan Offset Y"=w655, "Scan Offset X"=w655, "FPGA VI Reference"=w656) -> ()  [unwired: 6 in]
                        }
                        frame #1 {
                          n358 = Flush Queue(queue=w659) -> ()  [unwired: 1 in, 3 out]
                        }
                      }
                      n359 = global write "GlobalVars.vi" "Motor Movement Commant Sent"(FALSE ("Motor Movement Commant Sent")) -> ()
                    }
                  }
                }
              }
              n360 = global read "GlobalVars.vi" "Scanning"() -> (w636:bool)
              n361 = call <vilib>:"Release Semaphore.vi"("error in (no error)"=w628, "semaphore"=w630) -> ()  [unwired: 4 in, 2 out]
            }
            n362 = Initialize Array "Position Accumulator"(0.0, 3 ("dimension size")) -> (w621:dbl[])
            n363 = while "Update AOD/Motor Positions, Write Motor Position Information to File" {
              tunnel: w625 -> [w708]
              shift-right: [w706] -> _
              shift-left: w627 -> [w707]
              tunnel: w619 -> [w705]
              shift-right: [w691] -> _
              shift-left: w626 -> [w682]
              shift-right: [w694] -> _
              shift-left: w621 -> [w684]
              shift-right: [w693] -> _
              shift-left: w624 -> [w695]
              tunnel: w620 -> [w692]
              stop <- w709 continue-if-true
              n364 = case shown="False" "Reset AOD Cum Offsets" {
                tunnel: w682 -> [w710 w713]
                tunnel: [w710 w711] -> w681
                frame False {
                }
                frame True {
                  n365 = Multiply(x=w713, y=0.0) -> (x*y=w711:dbl[])
                }
              }
              n366 = local read "globals_semaphore"() -> (w699:T1)
              n367 = call <vilib>:"Acquire Semaphore.vi"("semaphore"=w699) -> ("error out"=w703:errorcluster, "semaphore out"=w704:T1)  [unwired: 4 in, 1 out]
              n368 = case shown="True" TRUE {
                tunnel: w708 -> [_ w744]
                tunnel: w707 -> [w719 w743]
                tunnel: [w719 w742] -> w706
                tunnel: w705 -> [_ w721]
                tunnel: w681 -> [w718 w740]
                tunnel: [w718 w739] -> w691
                tunnel: w704 -> [w717 w729]
                tunnel: w703 -> [w716 w728]
                tunnel: [w717 w729] -> w701
                tunnel: [w716 w728] -> w702
                tunnel: w695 -> [w715 w725]
                tunnel: w684 -> [w714 w724]
                tunnel: [w714 w723] -> w694
                tunnel: [w715 w722] -> w693
                tunnel: w692 -> [_ w720]
                frame False {
                }
                frame True {
                  n369 = global read "GlobalVars.vi" "AODPositionUpdateTime"() -> (w732:dbl)
                  n370 = global read "GlobalVars.vi" "MovementDetectionTime"() -> (w731:dbl)
                  n371 = Get Date/Time In Seconds() -> (seconds since 1Jan1904=w736:timestamp)
                  n372 = To Double Precision Float(number=w736) -> (double precision float=w735:dbl)
                  n373 = Subtract(x=w735, y=w732) -> (x-y=w741:dbl)
                  n374 = global read "GlobalVars.vi" "MovementSignal"() -> (w733:dbl[])
                  n375 = Greater?(x=w741, y="AOD Correction Refractory Time") -> (0:w726:bool)
                  n376 = feedback #2(0.0 ("Double")) -> (w737:dbl)
                  n377 = Not Equal?(x=w731, y=w737) -> (x != y?=w727:bool)
                  n378 = feedback-in #2(w731) -> ()
                  n379 = case "Tracking by Motor or Motor and AOD" shown="True" "Motion Tracking" {
                    tunnel: w744 -> [w750 w773]
                    tunnel: w743 -> [w751 w776]
                    tunnel: [w749 w774] -> w742
                    tunnel: w733 -> [w752 w777]
                    tunnel: w721 -> [_ w775]
                    tunnel: w740 -> [w753 w772]
                    tunnel: [w753 w771] -> w739
                    tunnel: w727 -> [w748 w764]
                    tunnel: w726 -> [_ w769]
                    tunnel: w725 -> [w747 w768]
                    tunnel: w724 -> [w746 w767]
                    tunnel: [w746 w766] -> w723
                    tunnel: [w747 w765] -> w722
                    tunnel: w720 -> [w745 w763]
                    frame False {
                      n380 = case shown="True" w748 {
                        tunnel: w752 -> [_ w756]
                        tunnel: w751 -> [w754 w762]
                        tunnel: w750 -> [_ w760]
                        tunnel: [w754 w758] -> w749
                        tunnel: w745 -> [_ w755]
                        frame False {
                        }
                        frame True {
                          n381 = Flush Queue(queue=w755) -> ()  [unwired: 1 in, 3 out]
                          n382 = Get Date/Time In Seconds() -> (seconds since 1Jan1904=w761:timestamp)
                          n383 = shared-variable "My Computer\\SutterShared.lvlib\\TargetPosition"(w756) -> ()  [unwired: 1 in, 1 out]
                          n384 = To Double Precision Float(number=w761) -> (double precision float=w757:dbl)
                          n385 = Add(x=w762, y=w756) -> (x+y=w758:dbl[])
                          n386 = Build Array (concatenate)(w757, w756) -> (w759:dbl[])
                          n387 = call "WriteMotorCorrectionData.vi"("Motion Correction Data"=w759, "AODAcq in"=w760) -> ()  [unwired: 8 in, 2 out]
                        }
                      }
                    }
                    frame True {
                      n388 = And(x=w769, y=w764) -> (x .and. y?=w770:bool)
                      n389 = case "Is AOD Refractory Period Over ?" shown="True" w770 {
                        tunnel: w777 -> [w783 w800]
                        tunnel: w776 -> [w784 w806]
                        tunnel: w775 -> [_ w811]
                        tunnel: [w784 w805] -> w774
                        tunnel: w773 -> [_ w809]
                        tunnel: w772 -> [w785 w797]
                        tunnel: [w785 w807] -> w771
                        tunnel: w768 -> [w780 w802]
                        tunnel: w767 -> [w782 w794]
                        tunnel: [w781 w793] -> w766
                        tunnel: [w779 0] -> w765
                        tunnel: w764 -> [_ _]
                        tunnel: w763 -> [_ w796]
                        frame False {
                          # "Disable averaging for now"
                          n390 = case "Is it in refractory Period and Getting New Motion Information" shown="True" FALSE {
                            tunnel: w783 -> [w786 w792]
                            tunnel: w782 -> [_ w791]
                            tunnel: [w786 w790] -> w781
                            tunnel: w780 -> [w787 w789]
                            tunnel: [w787 w788] -> w779
                            frame False {
                            }
                            frame True {
                              n391 = Add(x=w792, y=w791) -> (x+y=w790:dbl[])
                              n392 = Increment(x=w789) -> (x+1=w788:i32)
                            }
                          }
                        }
                        frame True {
                          n393 = Divide(x=w794, y=w802) -> (x/y=w799:dbl[])
                          n394 = Equal To 0?(x=w802) -> (x = 0?=w801:bool)
                          n395 = Multiply(x=w794, y=0.0) -> (x*y=w793:dbl[])
                          n396 = Select(t=w800, s=w801, f=w799) -> (s? t:f=w798:dbl[])
                          n397 = Add(x=w797, y=w798) -> (x+y=w808:dbl[])
                          n398 = Absolute Value(x=w808) -> (abs(x)=w804:dbl[])
                          n399 = Greater?(x=w804, y="Motor Correction Threshold") -> (0:w813:bool[])
                          n400 = Or Array Elements(Boolean array=w813) -> (logical OR=w812:bool)
                          n401 = case "If cumulative aod correction above motor threshold, move motors and zero all aod cumulative offsets" shown="False" w812 {
                            tunnel: w808 -> [_ w888]
                            tunnel: w811 -> [w823 _]
                            tunnel: [w818 w891] -> w807
                            tunnel: w809 -> [_ w894]
                            tunnel: w806 -> [w822 w893]
                            tunnel: [w822 w892] -> w805
                            tunnel: w797 -> [w817 w889]
                            tunnel: w798 -> [w816 _]
                            tunnel: w804 -> [_ _]
                            tunnel: w796 -> [w814 _]
                            frame False {
                              n402 = Absolute Value(x=w816) -> (abs(x)=w815:dbl[])
                              n403 = Greater?(x=w815, y="AOD Correction Threshold") -> (0:w820:bool[])
                              n404 = Or Array Elements(Boolean array=w820) -> (logical OR=w819:bool)
                              n405 = case "Is aod correction above the correction threshold" shown="True" w819 {
                                tunnel: w823 -> [_ w847]
                                tunnel: w816 -> [_ w834]
                                tunnel: [w824 w837] -> w818
                                tunnel: w817 -> [w824 w836]
                                tunnel: w814 -> [_ w832]
                                frame False {
                                }
                                frame True {
                                n406 = Get Date/Time In Seconds() -> (seconds since 1Jan1904=w844:timestamp)
                                n407 = To Double Precision Float(number=w844) -> (double precision float=w843:dbl)
                                n408 = local read "Scan Settings (um)"() -> (w846:T2)
                                n409 = global write "GlobalVars.vi" "AODPositionUpdateTime"(w843) -> ()
                                n410 = local read "Scan Settings"() -> (w845:T2)
                                n411 = Multiply(x=w834, y="AOD Feedback Gain") -> (x*y=w831:dbl[])
                                n412 = call "MicronsToSetting.vi"("Scan Settings"=w845, "Scan Settings (um)"=w846, "Microns (X,Y,Z)"=w831) -> ("Setting"=w833:i32[])  [unwired: 8 in]
                                n413 = Index Array(array=w831, index #1=0 ("index"), index #2=1 ("index"), index #3=2 ("index")) -> (element #1=→"XOut um":dbl, element #2=→"YOut um":dbl, element #3=→"ZOut um":dbl)
                                n414 = To Long Integer(number=w833) -> (32bit integer=w839:i32[])
                                n415 = Index Array(array=w839, index #1=0 ("index"), index #2=1 ("index"), index #3=2 ("index")) -> (element #1=w841:i32, element #2=w842:i32, element #3=w840:i32)
                                n416 = case "Note: X and Y in motor corrdinates become Y and X in AOD coordinates, can be fixed later to become consistent" shown="True" "AOD Feedback" {
                                tunnel: w847 -> [_ w869]
                                tunnel: w842 -> [_ w870]
                                tunnel: w841 -> [_ w856]
                                tunnel: w840 -> [_ w874]
                                tunnel: [w851 w857] -> w837
                                tunnel: w836 -> [w851 w859]
                                tunnel: w831 -> [_ w858]
                                tunnel: w832 -> [_ w855]
                                frame False {
                                }
                                frame True {
                                n417 = Flush Queue(queue=w855) -> ()  [unwired: 1 in, 3 out]
                                n418 = global read "GlobalVars.vi" "MovementSignal"() -> (w854:dbl[])
                                n419 = Add(x=w859, y=w858) -> (x+y=w857:dbl[])
                                n420 = case shown="False" "Invert X" {
                                tunnel: [w878 w880] -> w865
                                tunnel: w856 -> [w878 w879]
                                frame False {
                                }
                                frame True {
                                n421 = Negate(x=w879) -> (-x=w880:i32)
                                }
                                }
                                "XOut" <- w865
                                n422 = case shown="False" "Invert Y" {
                                tunnel: [w881 w883] -> w863
                                tunnel: w870 -> [w881 w882]
                                frame False {
                                }
                                frame True {
                                n423 = Negate(x=w882) -> (-x=w883:i32)
                                }
                                }
                                "YOut" <- w863
                                n424 = case shown="False" "Invert Z" {
                                tunnel: w874 -> [w875 w877]
                                tunnel: [w875 w876] -> w860
                                frame False {
                                }
                                frame True {
                                n425 = Negate(x=w877) -> (-x=w876:i32)
                                }
                                }
                                "ZOut" <- w860
                                n426 = Multiply(x=w854, y=0.0) -> (x*y=w853:dbl[])
                                n427 = global write "GlobalVars.vi" "MovementSignal"(w853) -> ()
                                n428 = xnode "Read/Write Control"("FPGA VI Reference In"=w869) -> ("OutOffset.X"=w862:i32, "OutOffset.Y"=w864:i32, "OutOffset.Z"=w861:i32)  [unwired: 1 in, 2 out]
                                n429 = Add(x=w863, y=w862) -> (x+y=w868:i32)
                                n430 = Add(x=w865, y=w864) -> (x+y=w867:i32)
                                n431 = Add(x=w860, y=w861) -> (x+y=w866:i32)
                                n432 = xnode "Read/Write Control"("FPGA VI Reference In"=w869, "InOffset.X"=w868, "InOffset.Y"=w867, "InOffset.Z"=w866) -> ()  [unwired: 1 in, 2 out]
                                }
                                }
                                }
                              }
                            }
                            frame True {
                              n433 = flat-sequence {
                                tunnel: w888 -> [w896]
                                tunnel: w893 -> [w897]
                                tunnel: w894 -> [w898]
                                tunnel: [w898] -> w886
                                tunnel: [w897] -> w885
                                tunnel: [w896] -> w884
                                tunnel: [w901] -> w887
                                tunnel: w886 -> [w905]
                                tunnel: w885 -> [w902]
                                tunnel: w884 -> [w899]
                                tunnel: [w907] -> w892
                                tunnel: w887 -> [w907]
                                frame #0 {
                                n434 = global write "GlobalVars.vi" "Motor Movement Completed"(FALSE ("Motor Movement Completed")) -> ()
                                }
                                frame #1 {
                                n435 = shared-variable "My Computer\\SutterShared.lvlib\\TargetPosition"(w899) -> ()  [unwired: 1 in, 1 out]
                                n436 = Add(x=w902, y=w899) -> (x+y=w901:dbl[])
                                n437 = Get Date/Time In Seconds() -> (seconds since 1Jan1904=w904:timestamp)
                                n438 = To Double Precision Float(number=w904) -> (double precision float=w900:dbl)
                                n439 = global write "GlobalVars.vi" "AODPositionUpdateTime"(w900) -> ()
                                n440 = Build Array (concatenate)(w900, w899) -> (w903:dbl[])
                                n441 = call "WriteMotorCorrectionData.vi"("Motion Correction Data"=w903, "AODAcq in"=w905) -> ()  [unwired: 8 in, 2 out]
                                }
                                frame #2 {
                                n442 = global write "GlobalVars.vi" "Motor Movement Commant Sent"(TRUE ("Motor Movement Commant Sent")) -> ()
                                }
                              }
                              n443 = Multiply(x=0.0, y=w889) -> (x*y=w891:dbl[])
                            }
                          }
                        }
                      }
                    }
                  }
                }
              }
              n444 = global read "GlobalVars.vi" "GoMove Notifier"() -> (w698:refnum<notifier>)
              n445 = call <vilib>:"Release Semaphore.vi"("error in (no error)"=w702, "semaphore"=w701) -> ("error out"=w697:errorcluster)  [unwired: 4 in, 1 out]
              n446 = Index Array(array=w691, index #1=0 ("index"), index #2=1 ("index"), index #3=2 ("index")) -> (element #1=→"Cum AOD Offset Y":dbl, element #2=→"Cum AOD Offset X":dbl, element #3=→"Cum AOD Offset Z":dbl)
              n447 = Send Notification(notification="READYTOMOVE", notifier=w698, error in (no error)=w697) -> ()  [unwired: 2 out]
              n448 = global read "GlobalVars.vi" "Scanning"() -> (w709:bool)
            }
          }
        }
        n449 = local write "Recording File"(w597) -> ()
        n450 = call-dynamic "Read Loop.vi"("error in (no error)"=w593, "ReadElements"=w612, "Queues"=w611, "AODAcq in"=w545) -> ("error out"=w543:errorcluster, "AODAcq out"=w544:refnum<class "AODAcq.lvclass">)  [unwired: 6 in]
        n451 = To Long Integer(number=w571) -> (32bit integer=w570:i32[][])
        n452 = flat-sequence {
          tunnel: w543 -> [w980]
          tunnel: [w980] -> w568
          frame #0 {
            n453 = local write "Finished"(TRUE ("Finished")) -> ()
          }
        }
        n454 = while {
          tunnel: w576 -> [_]
          tunnel: w573 -> [w1017]
          tunnel: w574 -> [_]
          tunnel: w542 -> [w991]
          tunnel: w608 -> [w1029]
          tunnel: w607 -> [_]
          tunnel: w606 -> [w1023]
          tunnel: w540 -> [w1026]
          tunnel: w558 -> [w1021]
          tunnel: w579 -> [w1022]
          shift-right: [w989] -> _
          shift-left: i64 0 -> [w1018]
          tunnel: w577 -> [w1019]
          tunnel: w570 -> [w1006]
          shift-right: [1] -> _
          shift-left: 0 -> [w987]
          i -> [w988]
          stop <- w1024 stop-if-true
          w1009 = 1000 ("length")
          n455 = Dequeue Element(queue=w1029, timeout in ms (-1)=w1017) -> (element=w982:waveform(i32)[])  [unwired: 1 in, 3 out]
          n456 = Square(x=w1023) -> (x^2=w1020:u16)
          n457 = local read "Finished"() -> (w1027:bool)
          n458 = xnode "Read/Write Control"("FPGA VI Reference In"=w991, "Control.Abort"="Abort") -> ()  [unwired: 1 in, 2 out]
          n459 = Divide(x=w1021, y=w1020) -> (x/y=w1016:dbl)
          n460 = Multiply(x=w1018, y=w1009) -> (x*y=w1011:i64)
          n461 = shared-variable "My Computer\\AODAcq.lvclass\\ReadFraction"() -> (w1030:dbl)  [unwired: 1 in, 1 out]
          n462 = shared-variable "My Computer\\AODAcq.lvclass\\ScanFraction"() -> (w996:dbl)  [unwired: 1 in, 1 out]
          "ScanProgress" <- w996
          n463 = Array Subset(array=w1019, index (row)=w1011, length (row)=w1009) -> (w1010:dbl[][])  [unwired: 2 in]
          n464 = Divide(x=w1016, y=2.0) -> (x/y=w1014:dbl)
          n465 = Not Equal To 0?(x=w988) -> (x != 0?=w1028:bool)
          n466 = Greater?(x=w996, y="Onset (fraction)") -> (0:w998:bool)
          n467 = Greater?(x=w996, y="Offset (fraction)") -> (0:w992:bool)
          n468 = Round Toward +Infinity(x=w1014) -> (ceil(x): smallest int >= x=w1013:dbl)
          n469 = local write "Progress"(w1030) -> ()
          n470 = Reshape Array(w1010, w1009) -> (w1008:dbl[])
          n471 = case shown="True" "Set AOD Scan Offset" {
            tunnel: w991 -> [_ w1056]
            frame False {
            }
            frame True {
              n472 = local read "Scan Settings (um)"() -> (w1051:T2)
              n473 = local read "Scan Settings"() -> (w1052:T2)
              n474 = case shown="False" "Add" {
                tunnel: w1056 -> [w1062 w1067]
                tunnel: w1051 -> [w1061 _]
                tunnel: "Scan Offset X" -> [w1060 w1066]
                tunnel: "Scan Offset Y" -> [w1059 w1065]
                tunnel: "Scan Offset Z" -> [w1058 w1064]
                tunnel: w1052 -> [w1057 w1063]
                tunnel: w1051 -> [_ w1068]
                frame False {
                  n475 = call "Set AOD Scanning Offsets.vi"("Scan Settings"=w1057, "Scan Settings (um)"=w1061, "Scan Offset Z"=w1058, "Scan Offset Y"=w1059, "Scan Offset X"=w1060, "FPGA VI Reference"=w1062) -> ()  [unwired: 6 in]
                }
                frame True {
                  n476 = call "Add AOD Scanning Offsets.vi"("Scan Settings"=w1063, "Scan Settings (um)"=w1068, "Scan Offset Z"=w1064, "Scan Offset Y"=w1065, "Scan Offset X"=w1066, "FPGA VI Reference"=w1067) -> ()  [unwired: 6 in]
                }
              }
            }
          }
          n477 = And(x=w1027, y=w1028) -> (x .and. y?=w1024:bool)
          n478 = case shown="True" "Average Motion Channels" {
            tunnel: w982 -> [w1035 w1042]
            tunnel: [w1032 w1038] -> w981
            frame False {
              n479 = Decrement(x="Motion Channel To Analyze") -> (x-1=w1033:i32)
              n480 = Index Array(array=w1035, index=w1033) -> (element=w1036:waveform(i32))
              n481 = Unbundle By Name(w1036) -> ("Y"=w1032:i32[])
            }
            frame True {
              n482 = for {
                tunnel: w1042 -> [w1046] mode=indexing
                shift-right: [w1043] -> w1041
                shift-left: i32[] [] ("Y") -> [w1044]
                n483 = Unbundle By Name(w1046) -> ("Y"=w1045:i32[])
                n484 = Add(x=w1045, y=w1044) -> (x+y=w1043:i32[])
              }
              n485 = Array Size(array=w1042) -> (size(s)=w1040:i32)
              n486 = Divide(x=w1041, y=w1040) -> (x/y=w1039:dbl[])
              n487 = To Long Integer(number=w1039) -> (32bit integer=w1038:i32[])
            }
          }
          n488 = And(x="Auto Recentering", y=w998) -> (x .and. y?=w997:bool)
          n489 = And(x="Auto Recentering", y=w992) -> (x .and. y?=w994:bool)
          n490 = Decrement(x=w1013) -> (x-1=w1012:dbl)
          n491 = To Long Integer(number=w1008) -> (32bit integer=w1007:i32[])
          n492 = case shown="True" w997 {
            frame False {
            }
            frame True {
              n493 = shared-variable "My Computer\\BehaviorShared.lvlib\\PauseBehavior"(TRUE ("PauseBehavior")) -> ()  [unwired: 1 in, 1 out]
            }
          }
          n494 = case shown="True" w994 {
            frame False {
            }
            frame True {
              n495 = shared-variable "My Computer\\BehaviorShared.lvlib\\PauseBehavior"(FALSE ("PauseBehavior")) -> ()  [unwired: 1 in, 1 out]
            }
          }
          n496 = Not(x=w1024) -> (.not. x?=w1025:bool)
          n497 = global write "GlobalVars.vi" "Scanning"(w1025) -> ()
          n498 = local read "Invert Intensity"() -> (w985:bool)
          n499 = case shown="False" w985 {
            tunnel: w981 -> [w1047 w1049]
            tunnel: [w1047 w1048] -> w984
            frame False {
            }
            frame True {
              n500 = Negate(x=w1049) -> (-x=w1048:i32[])
            }
          }
          n501 = call "Motion FIFO.vi"("Packet Length"=w1021, "Data"=w984, "Motion FIFO"=w1022) -> ("Number of Packets"=w1003:i32, "Array"=w1005:i32[])  [unwired: 7 in]
          n502 = Select(t=w1007, s="Simulated Motion Signal", f=w1005) -> (s? t:f=w1004:i32[])
          n503 = Select(t=1, s="Simulated Motion Signal", f=w1003) -> (s? t:f=w1001:i32)
          n504 = for {
            N: w1001 -> [_]
            tunnel: w1026 -> [w1098]
            tunnel: w1023 -> [w1085]
            tunnel: w1004 -> [w1097]
            tunnel: w1021 -> [w1094]
            tunnel: w1020 -> [_]
            tunnel: w1018 -> [w1092]
            tunnel: w1012 -> [w1088]
            tunnel: w1006 -> [w1082]
            tunnel: "Simulated Motion Signal" -> [w1081]
            tunnel: [w1072] -> w989
            tunnel: w987 -> [w1071]
            i -> [w1091]
            w1087 = 1 ("length")
            n505 = Multiply(x=w1094, y=w1091) -> (x*y=w1096:i32)
            n506 = local read "Number of Motion Volumes"() -> (w1078:i32)
            n507 = Array Subset "Select Packet"(array=w1097, index=w1096, length=w1094) -> (w1076:i32[])
            n508 = Array Size(array=w1076) -> (size(s)=w1079:i32)
            n509 = Divide(x=w1079, y=w1078) -> (x/y=w1073:dbl)
            n510 = Array Subset "Select First Motion Volume"(array=w1076, index=0, length=w1073) -> (w1074:i32[])
            n511 = Reshape Array(w1074, w1085, w1085, w1085) -> (w1089:i32[][][])
            n512 = Array Size(array=w1074) -> (size(s)=w1075:i32)
            n513 = Array Subset(array=w1089, index (dim 2)=w1088, length (dim 2)=w1087) -> (w1090:i32[][][])  [unwired: 4 in]
            n514 = Array Subset(array=w1089, index (dim 0)=w1088, length (dim 0)=w1087) -> (w1086:i32[][][])  [unwired: 4 in]
            n515 = Reshape Array(w1074, w1075, 1 ("dimension size")) -> (w1093:i32[][])
            n516 = case shown="True" "Motion Analysis" {
              tunnel: w1098 -> [_ w1136]
              tunnel: w1093 -> [_ w1130]
              tunnel: w1085 -> [_ w1131]
              tunnel: w1092 -> [w1103 w1111]
              tunnel: w1091 -> [_ w1126]
              tunnel: w1082 -> [_ w1120]
              tunnel: w1081 -> [_ w1119]
              tunnel: w1073 -> [_ w1113]
              tunnel: [w1103 w1110] -> w1072
              tunnel: w1071 -> [_ w1109]
              frame False {
                n517 = global read "GlobalVars.vi" "VI Open"() -> (w1104:bool)
                n518 = case shown="True" w1104 {
                  frame False {
                  }
                  frame True {
                    n519 = flat-sequence {
                      frame #0 {
                        n520 = global write "GlobalVars.vi" "VI Open"(FALSE ("VI Open")) -> ()
                      }
                      frame #1 {
                        n521 = Wait (ms)(milliseconds to wait=u32 100) -> ()  [unwired: 1 out]
                      }
                      frame #2 {
                        n522 = vi-ref "RunDuringExperiment.vi"() -> (w1107:refnum<vi>)
                        n523 = invoke on="Invoke Node" class="VI" method="Abort VI"(reference=w1107) -> (reference out=w1108:refnum<vi>)  [unwired: 2 in, 2 out]
                        n524 = invoke class="VI" method="FP.Close"(reference=w1108) -> ()  [unwired: 2 in, 3 out]
                      }
                    }
                  }
                }
              }
              frame True {
                n525 = Equal To 0?(x=w1126) -> (x = 0?=w1125:bool)
                n526 = Equal To 0?(x=w1109) -> (x = 0?=w1124:bool)
                n527 = Increment(x=w1111) -> (x+1=w1110:i64)
                n528 = global read "GlobalVars.vi" "VI Open"() -> (w1135:bool)
                n529 = local read "X-Y Motion Points"() -> (w1118:i32[][])
                n530 = local read "Y-Z Motion Points"() -> (w1115:i32[][])
                n531 = And(x=w1125, y=w1124) -> (x .and. y?=w1123:bool)
                n532 = case shown="False" w1135 {
                  frame False {
                    n533 = vi-ref "RunDuringExperiment.vi"() -> (w1137:refnum<vi>)
                    n534 = invoke on="Invoke Node" class="VI" method="FP.Open"(reference=w1137) -> (reference out=w1140:refnum<vi>)  [unwired: 4 in, 4 out]
                    n535 = invoke class="VI" method="Run VI"(reference=w1140, "Wait until done"=FALSE ("Wait Until Done"), "Auto Dispose Ref"=TRUE ("Auto Dispose Reference")) -> ()  [unwired: 2 in, 5 out]
                  }
                  frame True {
                  }
                }
                n536 = local read "Scan Settings (um)"() -> (w1133:T2)
                n537 = Array Subset(array=w1118, index (row)=0 ("index"), length (row)=w1113) -> (w1116:i32[][])  [unwired: 2 in]
                n538 = Array Subset(array=w1115, index (row)=0 ("index"), length (row)=w1113) -> (w1112:i32[][])  [unwired: 2 in]
                n539 = local read "Scan Settings"() -> (w1134:T2)
                n540 = Insert Into Array(array=w1116, new element=w1112) -> (w1122:i32[][])  [unwired: 2 in]
                n541 = Select(t=w1120, s=w1119, f=w1122) -> (s? t:f=w1121:i32[][])
                n542 = Cluster To Array(cluster=w1133) -> (array=w1128:i32[])
                n543 = Cluster To Array(cluster=w1134) -> (array=w1129:i32[])
                n544 = Bundle By Name(cluster=T6 {"gridsize"=0, "data"=[], "coordinates"=[], "settings"=[], "settings_um"=[], "needsreference"=FALSE}, "gridsize"=w1131, "data"=w1130, "coordinates"=w1121, "settings"=w1129, "settings_um"=w1128, "needsreference"=w1123) -> (w1127:T6)
                n545 = Lossy Enqueue Element(queue=w1136, element=w1127) -> ()  [unwired: 1 in, 4 out]
              }
            }
            n546 = Reshape Array(w1090, w1085, w1085) -> (w1083:i32[][])
            n547 = Reshape Array(w1086, w1085, w1085) -> (w1084:i32[][])
            n548 = Insert Into Array(array=w1083, new element=w1084) -> (w1095:i32[][])  [unwired: 2 in]
            n549 = local read "Motion Ch1"() -> (w1101:T5)
            n550 = To Single Precision Float(number=w1095) -> (single precision float=w1100:sgl[][])
            n551 = call "IMAQ ArrayToImage"("Image Pixels (Float)"=w1100, "Image"=w1101) -> ("Image Out"=w1102:T5)  [unwired: 8 in, 1 out]
            n552 = local write "Motion Ch1"(w1102) -> ()
          }
        }
      }
      frame 4 {
        n553 = call-dynamic "Reset.vi"("error in (no error)"=w1143, "AODAcq in"=w1144) -> ("error out"=w1142:errorcluster, "AODAcq out"=w1141:refnum<class "AODAcq.lvclass">)  [unwired: 8 in]
        n554 = call-dynamic "Read FPGA VI Reference.vi"("error in (no error)"=w1142, "AODAcq in"=w1141) -> ("error out"=w1150:errorcluster, "FPGA VI Reference"=w1151:T12, "AODAcq out"=w1149:refnum<class "AODAcq.lvclass">)  [unwired: 7 in]
        n555 = flat-sequence {
          tunnel: w1151 -> [w1154]
          tunnel: w1150 -> [w1152]
          tunnel: w1149 -> [w1153]
          tunnel: [w1153] -> w1146
          tunnel: [w1152] -> w1145
          tunnel: [w1156] -> w1147
          tunnel: [w1155] -> w1148
          tunnel: w1146 -> [w1158]
          tunnel: w1145 -> [w1157]
          frame #0 {
            n556 = call "SweepSettings.vi"("FPGA VI Reference Out"=w1154) -> ()  [unwired: 11 in]
          }
          frame #1 {
            n557 = call-dynamic "GetStatus.vi"("error in (no error)"=w1157, "AODAcq in"=w1158) -> ("error out"=w1156:errorcluster, "AODAcq out"=w1155:refnum<class "AODAcq.lvclass">)  [unwired: 7 in, 1 out]
          }
        }
      }
      frame 8 {
        n558 = Unbundle(w1169) -> ("queue out"=w1163:refnum<queue>)  [unwired: 3 out]
        n559 = local write "Ephys Acq"(FALSE ("Ephys")) -> ()
        n560 = local write "Ephys"(TRUE ("Ephys")) -> ()
        n561 = local write "Tab Control"(enum32{"Setup", "Volume", "Traces", "Motion"}."Traces" ("Tab Control")) -> ()
        n562 = call "DAQ Assistant"() -> ("task out"=w1170:refnum<k21>, "error out"=w1165:errorcluster)  [unwired: 16 in, 2 out]
        n563 = while {
          tunnel: w1170 -> [w1179]
          tunnel: w1163 -> [w1178]
          tunnel: [w1177] -> w1168
          tunnel: w1165 -> [w1176]
          tunnel: [w1174] -> w1164
          tunnel: [FALSE ("Ephys")] -> w1160
          stop <- w1180 stop-if-true
          n564 = call-poly <vilib>:"DAQmx Read.vi"("task/channels in"=w1179, "error in"=w1176) -> ("task out"=w1177:refnum<k21>, "data"=w1172:waveform(dbl), "error out"=w1175:errorcluster)  [unwired: 11 in]
          "Waveform Chart" <- w1172
          n565 = Build Array(w1172) -> (w1171:waveform(dbl)[])
          n566 = Enqueue Element(queue=w1178, element=w1171, error in (no error)=w1175) -> (error out=w1174:errorcluster)  [unwired: 1 in, 2 out]
          n567 = local read "Abort"() -> (w1180:bool)
        }
        "Ephys" <- w1160
        n568 = call <vilib>:"DAQmx Clear Task.vi"("task in"=w1168, "error in"=w1164) -> ("error out"=w1166:errorcluster)  [unwired: 13 in]
      }
      frame 16 {
        n569 = call "File Dialog"("start path"=path "M:/", "prompt"="Please select the AOD volume to load...", "pattern (all files)"="*.h5") -> ("selected path"=w1185:path, "cancelled"=w1181:bool)  [unwired: 9 in, 2 out]
        n570 = case shown="False" w1181 {
          tunnel: w1188 -> [w1227 w1235]
          tunnel: [w1194 w1235] -> w1186
          tunnel: w1185 -> [w1193 _]
          frame False {
            n571 = call "ReadAODVolume.vi"("error in"=w1227, "FilePath"=w1193) -> ("error out"=w1206:errorcluster, "settings_um"=w1225:dbl[][])  [unwired: 8 in]
            n572 = Array Size(array=w1225) -> (size(s)=w1224:i32[])
            n573 = Multiply Array Elements(1:w1224) -> (0:w1223:i32)
            n574 = Reshape Array(w1225, w1223) -> (w1222:dbl[])
            n575 = Open/Create/Replace File(file path (use dialog)=path "c:/temp/volumedata.bin", error in=w1206) -> (refnum out=w1203:refnum<file>, error out=w1205:errorcluster)  [unwired: 4 in, 1 out]
            n576 = local read "Scan Settings (um)"() -> (w1226:T2)
            n577 = Index Array(array=w1222, index #1=0 ("index"), index #2=1 ("index"), index #3=2 ("index"), index #4=3 ("index"), index #5=4 ("index"), index #6=5 ("index"), index #7=6 ("index"), index #8=7 ("index"), index #9=8 ("index")) -> (element #1=w1212:dbl, element #2=w1211:dbl, element #3=w1199:dbl, element #4=w1210:dbl, element #5=w1198:dbl, element #6=w1197:dbl, element #7=w1209:dbl, element #8=w1208:dbl, element #9=w1189:dbl)
            n578 = Bundle By Name(cluster=w1226, "XStart"=w1212, "XEnd"=w1211, "XNum"=w1199, "YStart"=w1210, "YEnd"=w1198, "YNum"=w1197, "ZStart"=w1209, "ZEnd"=w1208, "ZNum"=w1189) -> (w1207:T2)
            n579 = Compound Arithmetic op=MULTIPLY(w1199, w1197, w1189) -> (w1196:dbl)
            n580 = Read from Binary File(5:0, 8:w1205, 9:T9."native, host order" ("byte order (0:big-endian, network order)"), 10:-1 ("count (1)"), 11:w1203) -> (0:w1191:errorcluster, 2:w1192:i32[], 3:w1195:refnum<file>)  [unwired: 1 in, 1 out]
            n581 = local write "Scan Settings (um)"(w1207) -> ()
            n582 = flat-sequence "Two Channels of AOD Volumes" {
              tunnel: w1196 -> [w1229]
              tunnel: w1192 -> [w1232]
              tunnel: w1191 -> [w1230]
              tunnel: [w1230] -> w1190
              frame #0 {
                n583 = Reshape Array(w1232, 2 ("dimension size"), w1229) -> (w1231:i32[][])
                n584 = global write "GlobalVars.vi" "VolumeData"(w1231) -> ()
              }
            }
            n585 = Close File(refnum=w1195, error in=w1190) -> (error out=w1194:errorcluster)  [unwired: 1 out]
            n586 = case shown="No Error" w1194 {
              frame No Error {
                w1233 = 1.0 ("Progress")
                n587 = local write "Progress"(w1233) -> ()
                n588 = local write "ScanProgress"(w1233) -> ()
                n589 = local write "Tab Control"(enum32{"Setup", "Volume", "Traces", "Motion"}."Volume" ("Tab Control")) -> ()
              }
              frame Error {
              }
            }
          }
          frame True {
          }
        }
      }
    }
    n590 = call <vilib>:"Release Semaphore.vi"("error in (no error)"=w281, "semaphore"=w282) -> ()  [unwired: 4 in, 2 out]
    n591 = case shown="0, Default" w277 {
      tunnel: w289 -> [w319 w323]
      tunnel: [w319 w322] -> w288
      tunnel: w287 -> [w318 w321]
      tunnel: [w318 w320] -> w286
      frame 0, Default {
      }
      frame 1, 2 {
        n592 = call-dynamic "Stop.vi"("error in (no error)"=w321, "AODAcq in"=w323) -> ("error out"=w320:errorcluster, "AODAcq out"=w322:refnum<class "AODAcq.lvclass">)  [unwired: 8 in]
      }
    }
    "AODAcq out" <- w288
    n593 = call-dynamic "Read FPGA VI Reference.vi"("error in (no error)"=w286, "AODAcq in"=w288) -> ("error out"=w292:errorcluster, "FPGA VI Reference"=w293:T12)  [unwired: 7 in, 1 out]
    n594 = xnode "Read/Write Control"("FPGA VI Reference In"=w293, "error in"=w292) -> ("error out"=w291:errorcluster, "Control.Abort"=w294:bool)  [unwired: 1 out]
    n595 = while {
      tunnel: w291 -> [w335]
      tunnel: [w336] -> w296
      tunnel: [w335] -> w295
      stop <- TRUE stop-if-true
      n596 = local write "Finished"(FALSE ("Finished")) -> ()
      n597 = local read "Selection"() -> (w336:u32)
    }
    n598 = case shown="0, Default" w296 {
      tunnel: w295 -> [w338 w344 w361]
      tunnel: [w338 w343 w360] -> w303
      tunnel: w294 -> [_ w339 w363]
      frame 0, Default {
        w337 = FALSE ("ForceVolumeScan")
        n599 = local write "ForcePointScan"(w337) -> ()
        n600 = local write "ForceVolumeScan"(w337) -> ()
      }
      frame 2 {
        n601 = local read "Auto Recentering"() -> (w342:bool)
        n602 = Not(x=w339) -> (.not. x?=w341:bool)
        n603 = And(x=w342, y=w341) -> (x .and. y?=w340:bool)
        n604 = case shown="True" w340 {
          tunnel: w344 -> [w346 w359]
          tunnel: [w346 w359] -> w343
          frame False {
            w345 = FALSE ("ForceVolumeScan")
            n605 = local write "ForcePointScan"(w345) -> ()
            n606 = local write "ForceVolumeScan"(w345) -> ()
          }
          frame True {
            n607 = local write "ForceVolumeScan"(TRUE ("ForceVolumeScan")) -> ()
            n608 = local write "ForcePointScan"(FALSE ("ForcePointScan")) -> ()
            n609 = local read "Scan Settings (um) Saved"() -> (w355:T2)
            n610 = local read "Scan Settings Saved"() -> (w350:T2)
            n611 = Bundle By Name(cluster=w355, "XNum"="XNum", "YNum"="YNum") -> (w356:T2)
            n612 = Unbundle By Name(w355) -> ("XNum"=w354:i32, "YNum"=w353:i32)
            n613 = Bundle By Name(cluster=w350, "XNum"="XNum", "YNum"="YNum") -> (w347:T2)
            n614 = Divide(x=w354, y="XNum") -> (x/y=→"x_scale":dbl)
            n615 = Divide(x=w353, y="YNum") -> (x/y=→"y_scale":dbl)
            n616 = local write "Scan Settings (um)"(w356) -> ()
            n617 = local write "Scan Settings"(w347) -> ()
          }
        }
      }
      frame 1 {
        n618 = local read "ForceVolumeScan"() -> (w362:bool)
        n619 = Not(x=w363) -> (.not. x?=w364:bool)
        n620 = And(x=w362, y=w364) -> (x .and. y?=w365:bool)
        n621 = case shown="True" w365 {
          tunnel: w363 -> [w368 _]
          tunnel: w362 -> [w367 _]
          tunnel: w361 -> [w366 w374]
          tunnel: [w366 w373] -> w360
          frame False {
            n622 = case shown="True" w368 {
              tunnel: w367 -> [_ w370]
              frame False {
              }
              frame True {
                n623 = case shown="True" w370 {
                  frame False {
                  }
                  frame True {
                    n624 = local write "ForceVolumeScan"(FALSE ("ForceVolumeScan")) -> ()
                    n625 = local read "Scan Settings (um) Saved"() -> (w371:T2)
                    n626 = local write "Scan Settings (um)"(w371) -> ()
                  }
                }
              }
            }
            n627 = local write "ForcePointScan"(FALSE ("ForcePointScan")) -> ()
          }
          frame True {
            n628 = stacked-sequence {
              tunnel: w374 -> [w393 _ _ _ _]
              tunnel: [w392 _ _ _ _] -> w373
              frame #0 {
                # "Assumes same 'Z\" resolution"
                n629 = local write "EventDone"(FALSE ("EventDone")) -> ()
                n630 = local read "Scan Settings (um) Saved"() -> (w394:T2)
                n631 = local read "Scan Settings (um)"() -> (w404:T2)
                n632 = Unbundle(w394) -> ("XStart"=w395:i32, "XEnd"=w396:i32, "XNum"=w397:i32, "YStart"=w398:i32, "YEnd"=w399:i32, "YNum"=w400:i32, "ZStart"=w401:i32, "ZEnd"=w402:i32, "ZNum"=w403:i32)
                n633 = Unbundle(w404) -> ("XStart"=w405:i32, "XEnd"=w406:i32, "XNum"=w407:i32, "YStart"=w408:i32, "YEnd"=w409:i32, "YNum"=w410:i32, "ZStart"=w411:i32, "ZEnd"=w412:i32, "ZNum"=w413:i32)
                n634 = global read "GlobalVars.vi" "VolumeData"() -> (w375:i32[][])
                n635 = Build Array(w395, w396, w397, w398, w399, w400, w401, w402, w403) -> (w391:i32[])
                n636 = Build Array(w405, w406, w407, w408, w409, w410, w411, w412, w413) -> (w390:i32[])
                n637 = script code="x = linspace(settings(1),settings(2),settings(3));\ny = linspace(settings(4),settings(5),settings(6));\nz = linspace(settings(7),settings(8),settings(9));\n\nox = linspace(osettings(1),osettings(2),osettings(3));\noy = linspace(osettings(4),osettings(5),osettings(6));\noz = linspace(osettings(7),osettings(8),osettings(9));\n\nstack = stack(1,:);\nstack = reshape(stack,numel(y),numel(x),numel(z));\n\nvolout = zeros( numel(oy), numel(ox), numel(oz)) ;\nfor ii=1:size(stack,3)\n    volout(:,:,ii) = imresize(squeeze(stack(:,:,ii)), [size(volout,1) size(volout,2)], 'nearest') ;\nend ;\n\nvolout = reshape(volout, 1, numel(oy)*numel(ox)*numel(oz)) ;"("??"=w393, "stack"=w375, "settings"=w390, "osettings"=w391) -> ("??"=w392:errorcluster, "volout"=w387:dbl[][])
                n638 = local read "Scan Settings Saved"() -> (w385:T2)
                n639 = local read "Contrast"() -> (w381:dbl)
                n640 = local read "Section"() -> (w377:dbl)
                n641 = To Long Integer(number=w387) -> (32bit integer=w386:i32[][])
                n642 = global write "GlobalVars.vi" "VolumeData"(w386) -> ()
                n643 = local read "ImCh1"() -> (w384:T5)
                n644 = local read "ImCh2"() -> (w383:T5)
                n645 = local read "Offset"() -> (w382:dbl)
                n646 = call "Convert to Dynamic Data2"("2D Array"=w386) -> ("Dynamic Data Type"=w388:dynamicdata)  [unwired: 3 in]
                n647 = local read "Mirror Ch1 Display"() -> (w379:bool)
                n648 = call "UpdateStack.vi"("Contrast"=w381, "Scan Settings"=w385, "Offset"=w382, "Section"=w377, "ImData"=w386, "Im2 2"=w383, "Im1 In"=w384) -> ("Im2 Out"=w389:T5, "Im1 Out"=w376:T5)  [unwired: 3 in]
                n649 = call "Create Histogram2"("Signal"=w388) -> ("Histogram"=w380:dynamicdata)  [unwired: 9 in, 1 out]
                n650 = local write "ImCh1"(w376) -> ()
                n651 = local write "Histogram"(w380) -> ()
                n652 = case shown="True" w379 {
                  tunnel: w376 -> [_ w417]
                  tunnel: [w415 w416] -> w378
                  tunnel: w389 -> [w415 w418]
                  frame False {
                  }
                  frame True {
                    n653 = call "IMAQ Copy"("Image Dst"=w418, "Image Src"=w417) -> ("Image Dst Out"=w416:T5)  [unwired: 4 in, 1 out]
                  }
                }
                n654 = local write "ImCh2"(w378) -> ()
              }
              frame #1 {
                n655 = local read "Scan Settings Saved"() -> (w419:T2)
                n656 = local read "Scan Settings (um) Saved"() -> (w420:T2)
                n657 = local write "Scan Settings"(w419) -> ()
                n658 = local write "Scan Settings (um)"(w420) -> ()
              }
              frame #2 {
                n659 = property on="Recenter" class="Bool (strict)"("Val(Sgnl)"=TRUE ("Value (Signaling)")) -> ()  [unwired: 2 in, 2 out]
              }
              frame #3 {
                n660 = while {
                  tunnel: [FALSE ("Value (Signaling)")] -> w422
                  stop <- w424 stop-if-true
                  n661 = local read "EventDone"() -> (w424:bool)
                }
                n662 = property on="Recenter" class="Bool (strict)"("Val(Sgnl)"=w422) -> ()  [unwired: 2 in, 2 out]
              }
              frame #4 {
                n663 = local write "ForceVolumeScan"(FALSE ("ForceVolumeScan")) -> ()
                n664 = local write "ForcePointScan"(TRUE ("ForcePointScan")) -> ()
                n665 = Wait (ms)(milliseconds to wait="Post Recentering Wait (ms)") -> ()  [unwired: 1 out]
              }
            }
          }
        }
      }
    }
    n666 = call <vilib>:"Simple Error Handler.vi"("error in (no error)"=w303) -> ()  [unwired: 4 in, 5 out]
    "Volume" <- "Volume Scan"
    "Scan" <- "Points Scan"
    "Numeric" <- w310
  }
  "Stopped" <- w21
  n667 = while {
    tunnel: w35 -> [w1238]
    stop <- w1237 stop-if-true
    n668 = local read "Tab Control"() -> (w1236:enum32{"Setup", "Volume", "Traces", "Motion"})
    n669 = case shown="\"Traces\"" w1236 {
      tunnel: w1238 -> [_ w1244]
      frame "Setup", Default {
        n670 = Wait (ms)(milliseconds to wait=u32 150) -> ()  [unwired: 1 out]
      }
      frame "Traces" {
        n671 = Dequeue Element(queue=w1244, timeout in ms (-1)=500) -> (element=w1241:waveform(dbl)[], timed out?=w1240:bool, error out=w1242:errorcluster)  [unwired: 1 in, 1 out]
        n672 = call <vilib>:"Clear Errors.vi"("error in (no error)"=w1242) -> ()  [unwired: 5 in, 2 out]
        n673 = case shown="False" w1240 {
          tunnel: w1241 -> [w1245 _]
          frame False {
            "Ephys Signals" <- w1245
          }
          frame True {
          }
        }
      }
    }
    n674 = local read "Stopped"() -> (w1237:bool)
  }
  n675 = case shown="True" w21 {
    tunnel: [errorcluster {"status"=FALSE, "code"=0, "source"=""} ("error out") w1248] -> w22
    frame False {
    }
    frame True {
      n676 = global read "GlobalVars.vi" "VI Open"() -> (w1247:bool)
      n677 = case shown="True" w1247 {
        tunnel: [errorcluster {"status"=FALSE, "code"=0, "source"=""} ("error out") w1250] -> w1248
        frame False {
        }
        frame True {
          n678 = flat-sequence {
            tunnel: [w1255] -> w1250
            frame #0 {
              n679 = global write "GlobalVars.vi" "VI Open"(FALSE ("VI Open")) -> ()
            }
            frame #1 {
              n680 = Wait (ms) "Allow VI to Stop"(milliseconds to wait=u32 100) -> ()  [unwired: 1 out]
            }
            frame #2 {
              n681 = vi-ref "RunDuringExperiment.vi"() -> (w1253:refnum<vi>)
              n682 = invoke class="VI" method="Abort VI"(reference=w1253) -> (reference out=w1254:refnum<vi>)  [unwired: 2 in, 2 out]
              n683 = invoke class="VI" method="FP.Close"(reference=w1254) -> (error out=w1255:errorcluster)  [unwired: 2 in, 2 out]
            }
          }
        }
      }
    }
  }
  n684 = stacked-sequence {
    tunnel: w22 -> [_ w1260]
    frame #0 {
      n685 = Wait Until Next ms Multiple(millisecond multiple=u32 500) -> ()  [unwired: 1 out]
    }
    frame #1 {
      n686 = disable-structure shown="Disabled" {
        disable-tunnel: w1260 -> [w1264 _]
        frame Disabled {
          n687 = global read "GlobalVars.vi" "MotionAnalysis"() -> (w1262:refnum<queue>)
          n688 = local read "Motion FIFO"() -> (w1263:refnum<queue>)
          n689 = Release Queue(queue=w1262, error in (no error)=w1264) -> (error out=w1261:errorcluster)  [unwired: 1 in, 2 out]
          n690 = Release Queue(queue=w1263, error in (no error)=w1261) -> ()  [unwired: 1 in, 3 out]
        }
        frame Enabled {
        }
      }
      n691 = local read "Scan Settings Saved"() -> (w1258:T2)
      n692 = global read "GlobalVars.vi" "GoMove Notifier"() -> (w1257:refnum<notifier>)
      n693 = local read "Scan Settings (um) Saved"() -> (w1259:T2)
      n694 = Release Notifier(notifier=w1257) -> ()  [unwired: 2 in, 3 out]
      n695 = local write "Scan Settings"(w1258) -> ()
      n696 = local write "Scan Settings (um)"(w1259) -> ()
    }
  }
  "Points_um" <- dbl[][] [] ("Points_um")
